vi "Demo HAL Tester v2.vi"() -> ()   [LabVIEW 2014]
uses:
  <vilib>/Utility/miscctls.llb/LVPointTypeDef.ctl
  <vilib>/Utility/miscctls.llb/LVRectTypeDef.ctl
  Typedefs/Driver Data.ctl
  Typedefs/HW Data.ctl
  TypeDefs/HAL Config Data.ctl
  DriverMasterSync/build/DriverMasterSync.lvlibp/Modules/HAL/DriverMasterSync/DriverMasterSyncClass/DriverMasterSync.lvclass
  DriverMasterAsync/builds/DriverMasterAsync.lvlibp/Modules/HAL/DriverMasterAsync/DriverMasterAsyncClass/DriverMasterAsync.lvclass
  <vilib>/Utility/miscctls.llb/LVRangeTypeDef.ctl
  APIs/Message Queue/Enqueue Message (Single).vi
  APIs/Message Queue/WINFAS 2 Message Queue.lvlib
  APIs/Data Queue/WINFAS 2 Data Queue.lvlib
  HWSyncLoop/HWSyncLoop.lvlib
  HWAsyncLoop/HWAsyncLoop.lvlib
  <vilib>/Utility/file.llb/Write To Spreadsheet File (string).vi
  <vilib>/Utility/file.llb/Read From Spreadsheet File (string).vi
  <vilib>/Utility/LVLibp/NI_PackedLibraryUtility.lvlib
panel:
  out "Enable Waveforms":u32
  out "HW Position":i32
  out "Display Tab":enum32{"Splash", "Sync", "Async"}(tab)
  out "Driver Name Sync 2":string
  out "Mensajes para Usuario (Síncronos)":string
  out "Sync DI":bool[][](array[boolean])
  out "Sync DO":bool[][](array[boolean])
  out "Encoder":sgl caption="Encoder:" format="%.1f"
  in  "Escala en mm:":enum32{"x0.25", "x0.5", "x1", "x2"}(radio)=enum."x1"
  out "Tabla TDX":string[][](table)
  out "Waveform Graph":sgl[][](graph)
  out "Mensajes para el usuario (Asíncronos)":string
  out "Tabla Med Async":string[][](table)
  out "Status Bar":string
  out "Command Tab":enum32{"Configuración", "Comandos"}(tab)
  in  "Descripción":string
  in  "Open Cfg":bool
  in  "Save Cfg":bool
  in  "New Cfg":bool
  in  "Driver Tree":string(tree)
  in  "HAL Activate":bool
  in  "Driver Unload":bool
  out "Last Mod":string caption="Última modificación:"
  out "Cfg Driver Name":string caption="Nombre:"
  in  "Cfg Panel Open":bool
  in  "Driver Load":bool
  in  "Dispositivos Conectados":i32(listbox)
  out "Sync/Async CMD":enum32{"Sync", "Async"}(tab)
  out "Estado:":string
  in  "Sync ACQ Start":bool
  in  "Output Control":bool[][](array[boolean])
  in  "Write Digital Out":bool
  in  "Zero Encoder":bool
  out "Driver Name Sync":string
  in  "Async ACQ":bool
  in  "Async Zero":bool
  in  "Async Action 2":bool
  in  "Async Action 1":bool
  out "Driver Name Async":string
  in  "HAL Deactivate":bool
  # "INSTRUCCIONES DE USO\n\n- Panel Configuración-\n1. Crear Nuevo Configuración o Abrir una ya existente (Los archivos de configuración tiene extensión \".config\"; Por ej \"CAP 16T.config\"). Puede guardar  sus propias\nconfiguraciones con el botón Guardar\n\n- Panel Driver -\n1. En la lista desplegable se pueden visualizar y seleccionar los 5 Procesos Síncronos (Sync#) y los 10 Procesos Asíncronos (Async#),\ncon su respectivo driver cargado (Por ej \"CAP-USB-1.lvlibp\")\n2. Una vez seleccionado un Proceso se puede cargar un Driver en el mismo mediante el boton \"\"Cargar Nuevo...\"\n3. Para acceder a su panel de configuración presione \"Configuración...\"\n4. Para eliminar le Driver cargado del proceso seleccionado presione \"Eliminar\"\n\n- CONECTAR -\n1. Una vez definida la configuración de Drivers que uno desea, al presionar \"Conectar >\" se establecerán conexiones con todos los dispositivos elegidos y se comenzará el proceso de\nadquisición en Auto-Refresh de los procesos Síncronos. VERIFIQUE QUE TODO EL CABLEADO ESTÉ CORRECTO, sino la aplicación devolverá error.\n\n- Panel Dispositivos Conectados -\n1. Una vez conectados los dispositivos se podrá seleccionar cada Dispositivo que esté funcionando y monitorear sus valores de adquisición, como así también darle comandos \npara que adquiera más datos, realice mediciones, escriba el encoder en Cero,escriba y lea salidas, etc.\n\n- DESCONECTAR -\n1. Una vez que desee terminar con la adquisición, debe presionar \"Desconectar >\". ASEGURESE QUE NINGÚN DISPOSITIVO ESTE EN ESTADO DE MEDICIÓN,\nsino la aplicación devolverá error."
  # "Medición de Transductores (TODOS)"
  # "Encoder y Entradas/Salidas Digitales"
  # "Entradas"
  # "1      2      3      4      5      6      7      8      9     10    11    12    13    14    15    16"
  # "17    18    19    20    21    22    23    24    25    26    27    28    29    30    31    32"
  # "Salidas"
  # "1      2      3      4      5      6      7      8      9     10    11    12    13    14    15    16"
  # "17    18    19    20    21    22    23    24    25    26    27    28    29    30    31    32"
  # "Valores medidos (Asíncronos)"
  # "Configuración"
  # "Conecta todos los dispositivos y comienza\nel ciclo de prueba"
  # "Driver Seleccionado"
  # "Comandos"
  # "(Dispositivo Midiendo = subrayado)"
  # "Medición"
  # "(Solo se permite de a un dispositivo por vez)"
  # "Salidas Digitales"
  # "Seleccione los estados de las salidas y presione\n\"Escribir Salidas\" para escribir el puerto entero"
  # "1      2      3      4      5      6      7      8      9     10    11    12    13    14    15    16"
  # "17    18    19    20    21    22    23    24    25    26    27    28    29    30    31    32"
  # "Encoder"
  # "Pone al encoder en valor 0 (Cero)"
  # "Acción"
  # "Medición"
  # "Realizo una medición asíncrona"
  # "Realiza Acción 1"
  # "Poner en Cero el Dispositivo"
  # "Realiza Acción 2"
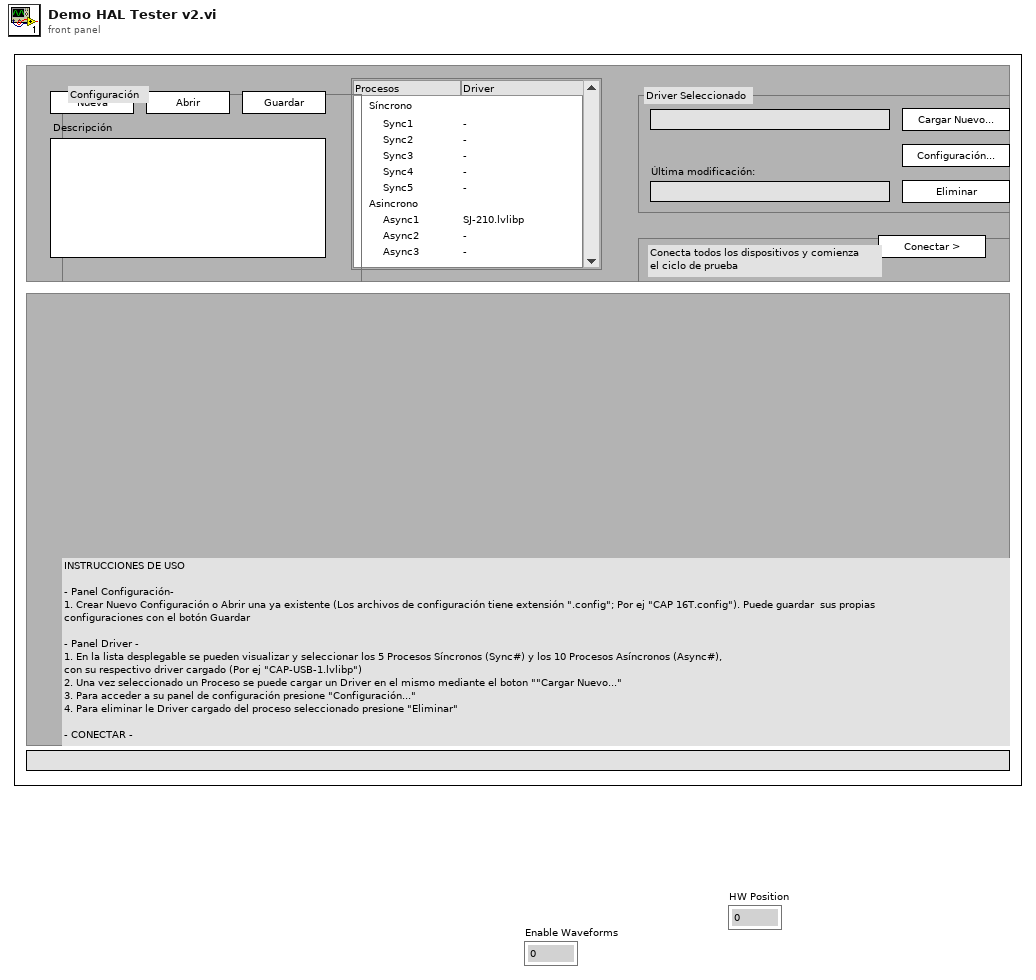
[diagram p1: front panel]
types:
  T1 = typedef "HAL Config Data.ctl" = cluster{"HWSync Index":u32, "Driver Name":string, "Channel Mask":u64}
  T2 = typedef "HW Data.ctl" = cluster{"Driver Name":string, "Sincrono?":bool, "HW Position":i32, "Busy?":bool}
  T3 = enum8{"Enabled", "Disabled", "Disabled and Grayed Out"}
  T4 = typedef "Driver Data.ctl" = cluster{"Dirección de Driver":path, "Config Data":variant}
  T5 = typedef "LVRectTypeDef.ctl" = cluster{"Left":i16, "Top":i16, "Right":i16, "Bottom":i16}
  T6 = typedef "LVPointTypeDef.ctl" = cluster{"Horizontal":i16, "Vertical":i16}
  T7 = typedef "WINFAS 2 Message Queue.lvlib/All Message Queues.ctl" = cluster{"CORE":refnum<queue>, "Event UI":refnum<queue>, "Display UI":refnum<queue>, "MATH":refnum<queue>, "SEQ":refnum<queue>, "DB":refnum<queue>, "ERR":refnum<queue>, "HAL":refnum<queue>, "HWSync1":refnum<queue>, "HWSync2":refnum<queue>, "HWSync3":refnum<queue>, "HWSync4":refnum<queue>, "HWSync5":refnum<queue>, "HWAsync1":refnum<queue>, "HWAsync2":refnum<queue>, "HWAsync3":refnum<queue>, "HWAsync4":refnum<queue>, "HWAsync5":refnum<queue>, "HWAsync6":refnum<queue>, "HWAsync7":refnum<queue>, "HWAsync8":refnum<queue>, "HWAsync9":refnum<queue>, "HWAsync10":refnum<queue>}
  T8 = typedef "WINFAS 2 Data Queue.lvlib/All Data Queues Cluster.ctl" = cluster{"Queues":cluster{"ACQ HWSync1":refnum<queue>, "ACQ HWSync2":refnum<queue>, "ACQ HWSync3":refnum<queue>, "ACQ HWSync4":refnum<queue>, "ACQ HWSync5":refnum<queue>}, "Notifiers":cluster{"Control":cluster{"CTRL HWSync1":refnum<notifier>, "CTRL HWSync2":refnum<notifier>, "CTRL HWSync3":refnum<notifier>, "CTRL HWSync4":refnum<notifier>, "CTRL HWSync5":refnum<notifier>}, "Acquisition":cluster{"ACQ HWSync1":refnum<notifier>, "ACQ HWSync2":refnum<notifier>, "ACQ HWSync3":refnum<notifier>, "ACQ HWSync4":refnum<notifier>, "ACQ HWSync5":refnum<notifier>}, "Async":cluster{"ACQ HWAsync1":refnum<notifier>, "ACQ HWAsync2":refnum<notifier>, "ACQ HWAsync3":refnum<notifier>, "ACQ HWAsync4":refnum<notifier>, "ACQ HWAsync5":refnum<notifier>, "ACQ HWAsync6":refnum<notifier>, "ACQ HWAsync7":refnum<notifier>, "ACQ HWAsync8":refnum<notifier>, "ACQ HWAsync9":refnum<notifier>, "ACQ HWAsync10":refnum<notifier>}}}
  T9 = enum16{"open", "replace", "create", "open or create", "replace or create", "replace or create with confirmation"}
  T10 = typedef "LVRangeTypeDef.ctl" = cluster{"Minimum":dbl, "Maximum":dbl, "Increment":dbl, "Minor Increment":dbl, "Start":dbl}
  T11 = cluster{"Dirección de Driver":path, "Config Data":variant}
  T12 = cluster{"Dirección de Driver":path, "Config Data":variant}[]
  T13 = cluster{"ACQ HWSync1":refnum<notifier>, "ACQ HWSync2":refnum<notifier>, "ACQ HWSync3":refnum<notifier>, "ACQ HWSync4":refnum<notifier>, "ACQ HWSync5":refnum<notifier>}
  T14 = cluster{"CTRL HWSync1":refnum<notifier>, "CTRL HWSync2":refnum<notifier>, "CTRL HWSync3":refnum<notifier>, "CTRL HWSync4":refnum<notifier>, "CTRL HWSync5":refnum<notifier>}
  T15 = cluster{"ACQ HWSync1":refnum<queue>, "ACQ HWSync2":refnum<queue>, "ACQ HWSync3":refnum<queue>, "ACQ HWSync4":refnum<queue>, "ACQ HWSync5":refnum<queue>}
  T16 = typedef "WINFAS 2 Data Queue.lvlib/Async Acquisition Data Cluster.ctl" = cluster{"Data":sgl[]}
  T17 = typedef "WINFAS 2 Data Queue.lvlib/Acquisition Data 1 Sample Cluster.ctl" = cluster{"TDX":sgl[], "Encoder":sgl}
  T18 = typedef "WINFAS 2 Data Queue.lvlib/Control Data Cluster.ctl" = cluster{"Encoder":sgl, "DI":bool[], "DO":bool[]}
  T19 = cluster{"HWSync1":refnum<queue>, "HWSync2":refnum<queue>, "HWSync3":refnum<queue>, "HWSync4":refnum<queue>, "HWSync5":refnum<queue>}
  T20 = cluster{"HWAsync1":refnum<queue>, "HWAsync2":refnum<queue>, "HWAsync3":refnum<queue>, "HWAsync4":refnum<queue>, "HWAsync5":refnum<queue>, "HWAsync6":refnum<queue>, "HWAsync7":refnum<queue>, "HWAsync8":refnum<queue>, "HWAsync9":refnum<queue>, "HWAsync10":refnum<queue>}
  T21 = enum32{"invalid app kind", "Development System", "Run Time System", "Student Edition", "Embedded LabVIEW", "Evaluation", "Custom"}
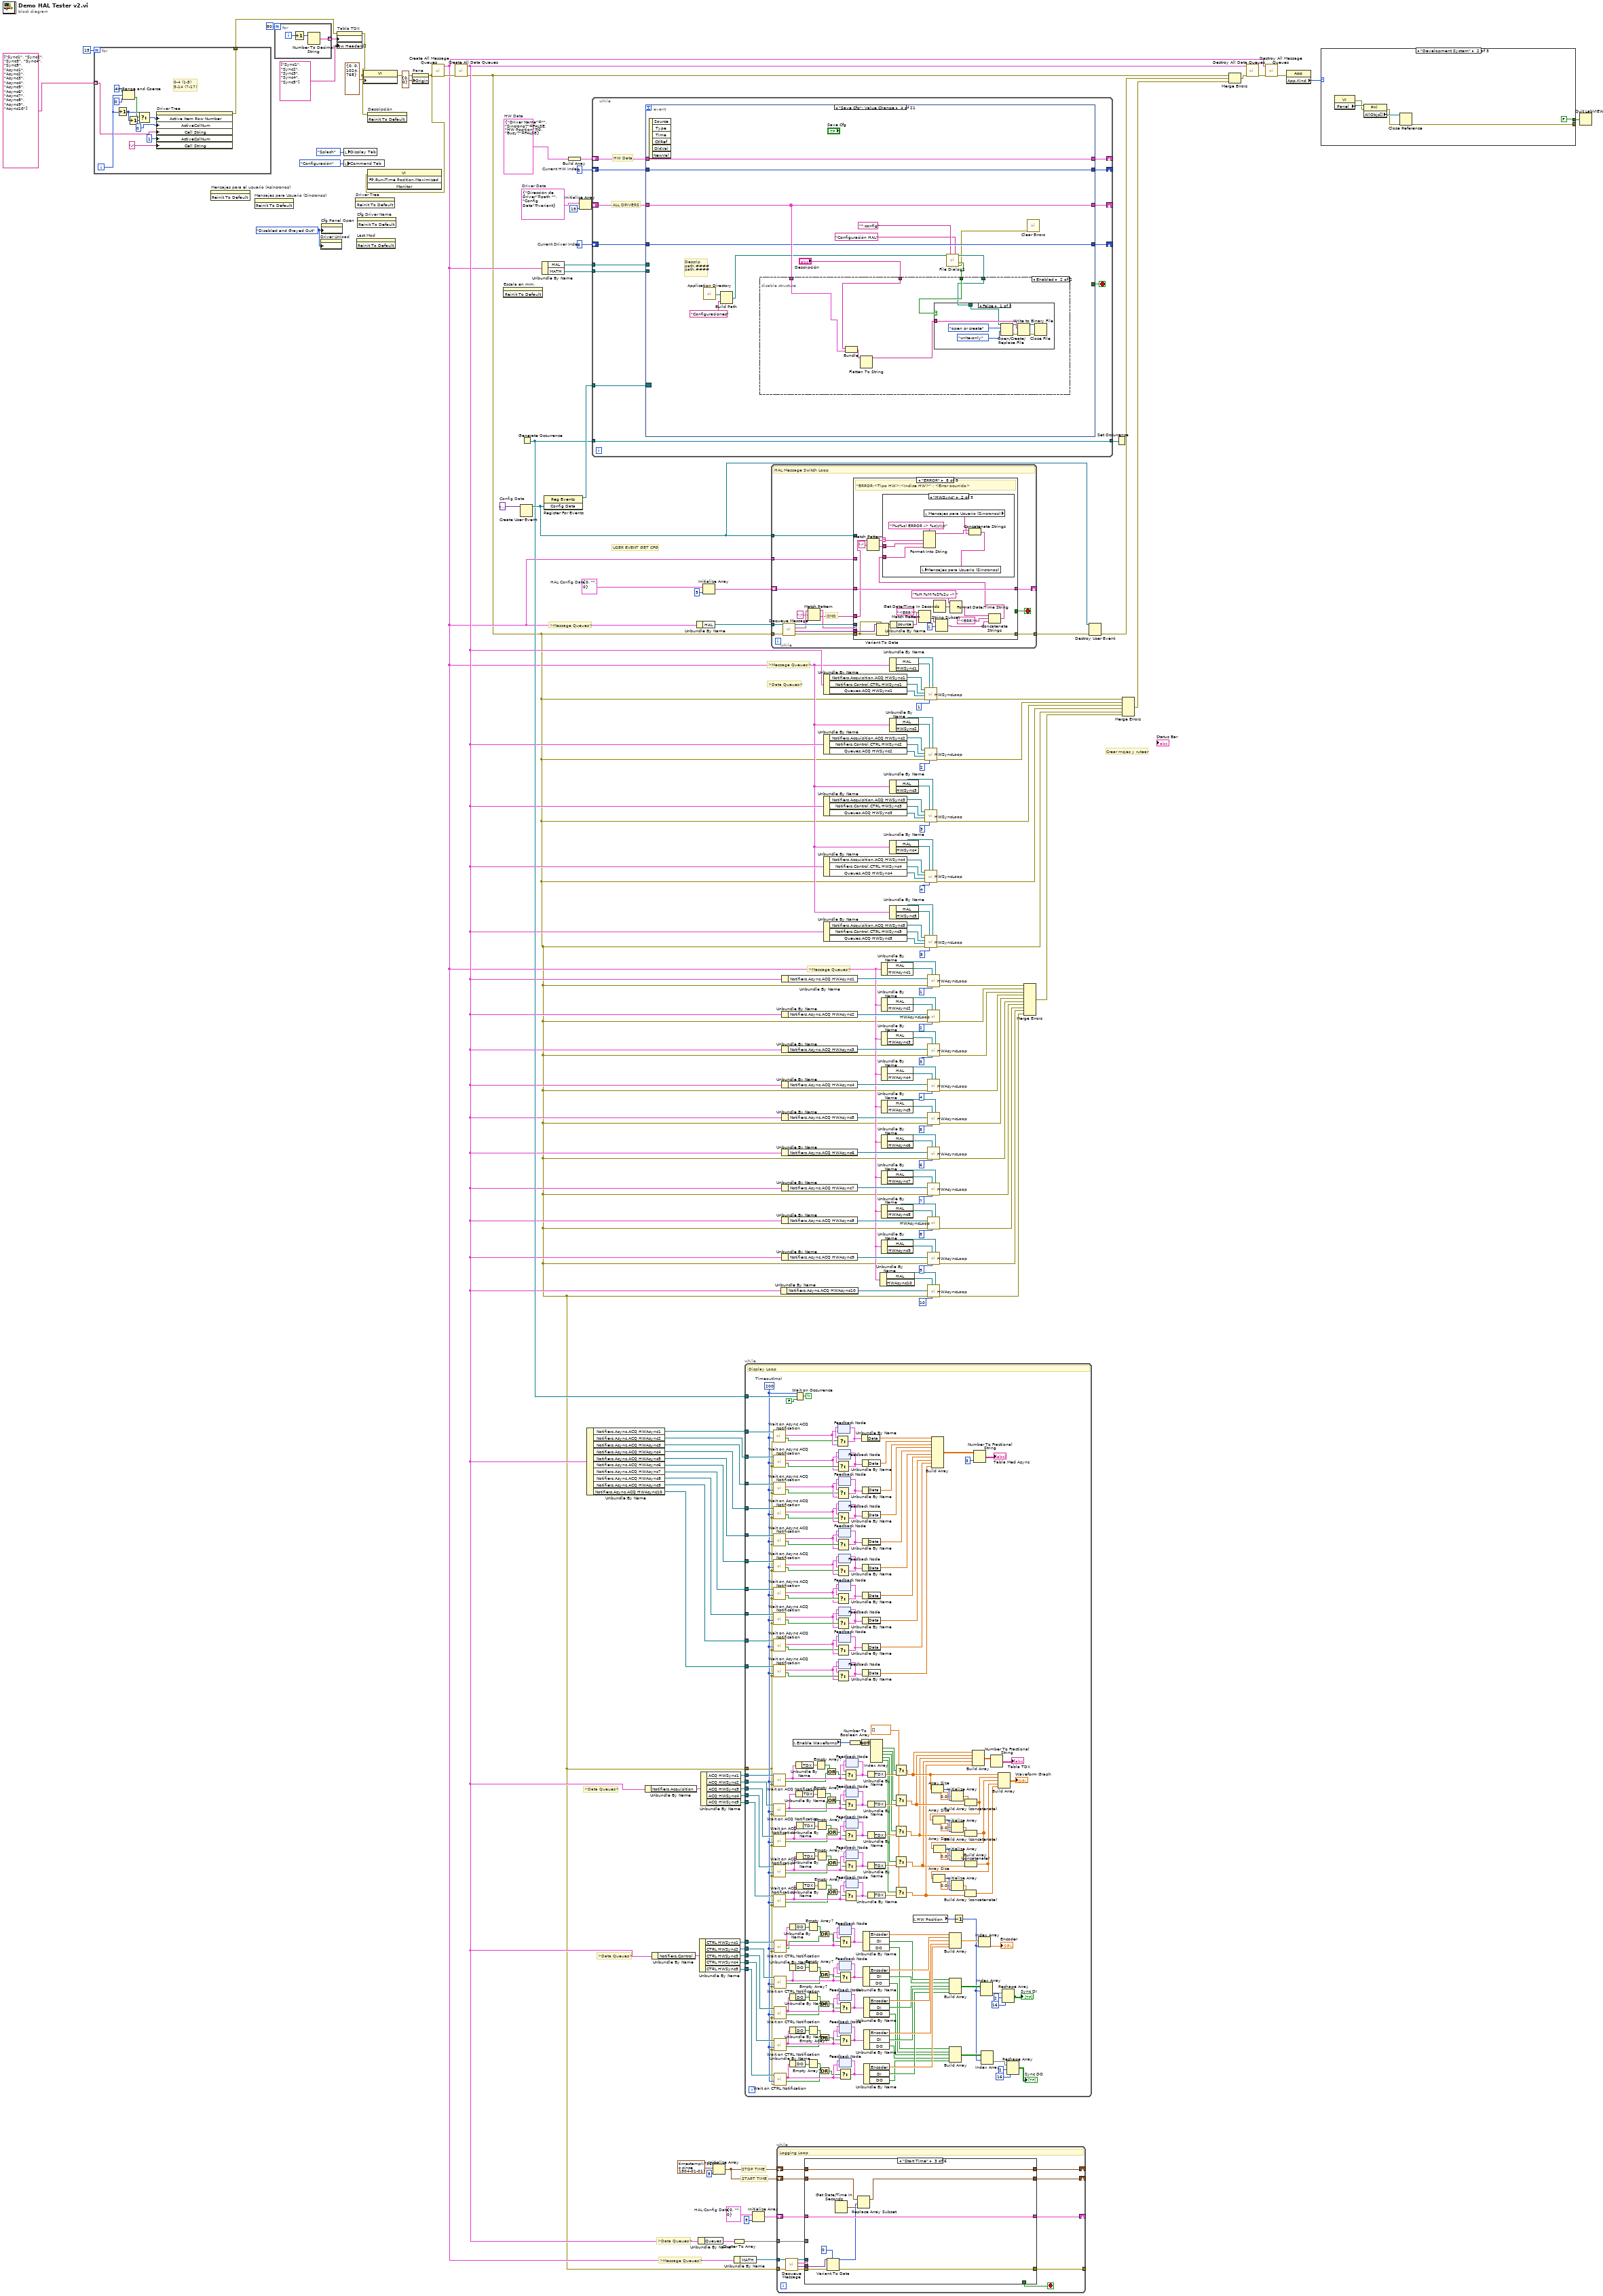
[diagram p0: block diagram]
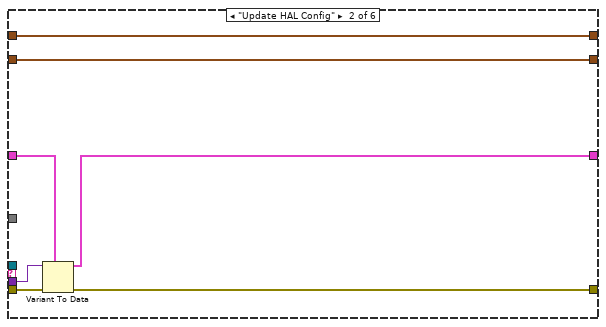
[diagram p3: hidden frame]
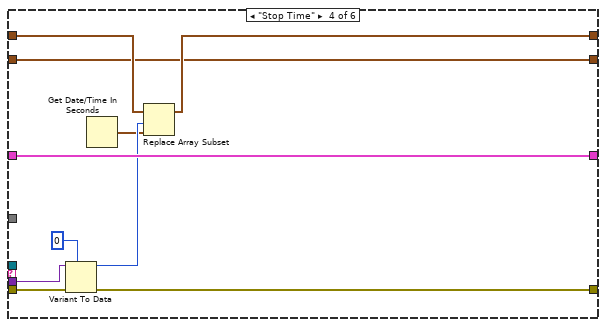
[diagram p4: hidden frame]
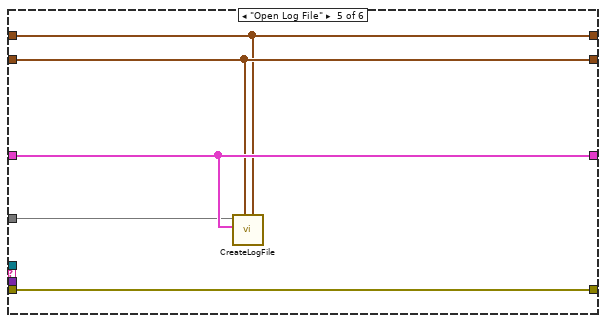
[diagram p5: hidden frame]
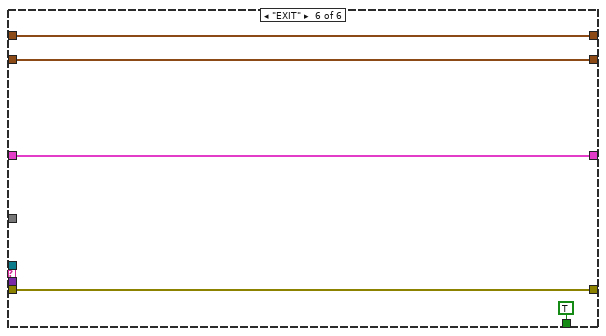
[diagram p6: hidden frame]
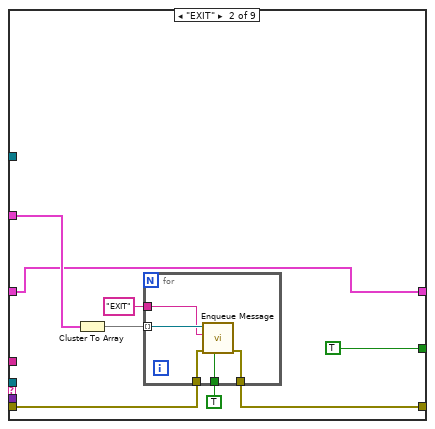
[diagram p8: hidden frame]
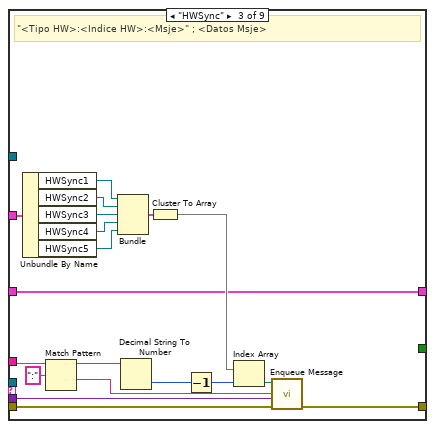
[diagram p9: hidden frame]
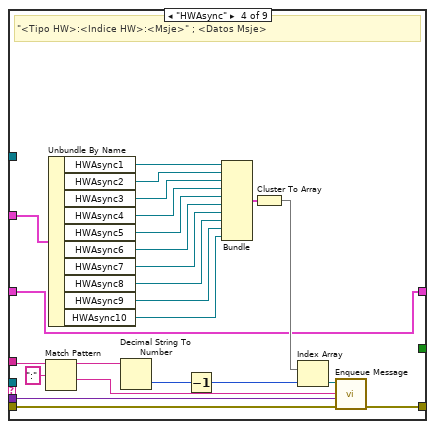
[diagram p10: hidden frame]
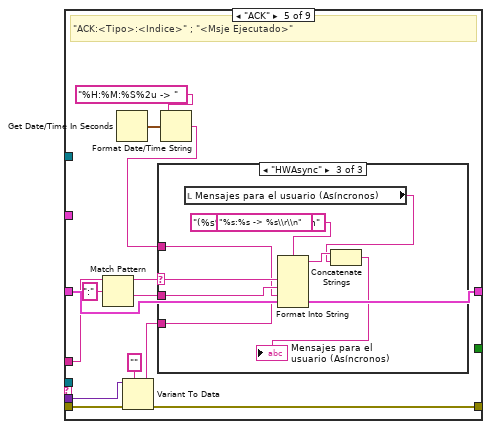
[diagram p11: hidden frame]
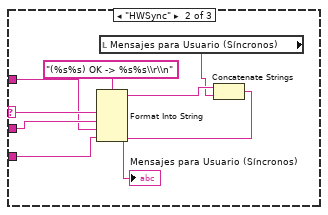
[diagram p13: hidden frame]
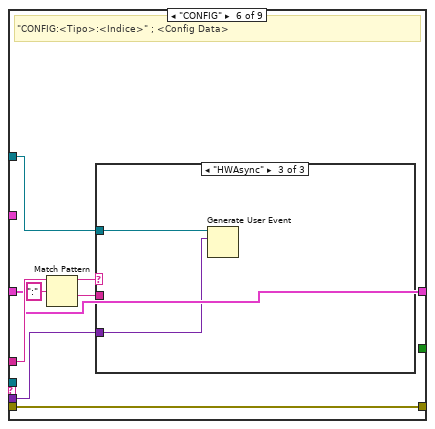
[diagram p14: hidden frame]
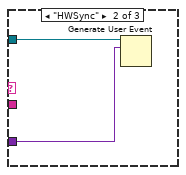
[diagram p16: hidden frame]
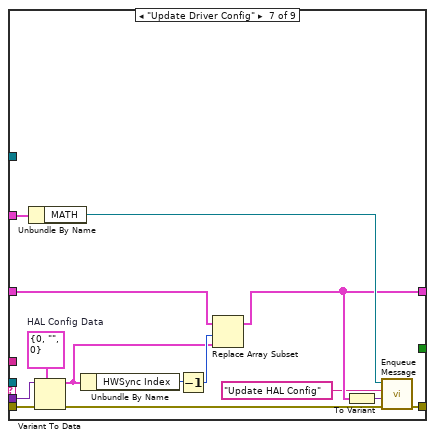
[diagram p17: hidden frame]
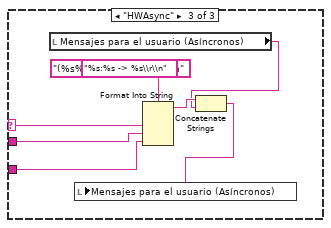
[diagram p19: hidden frame]
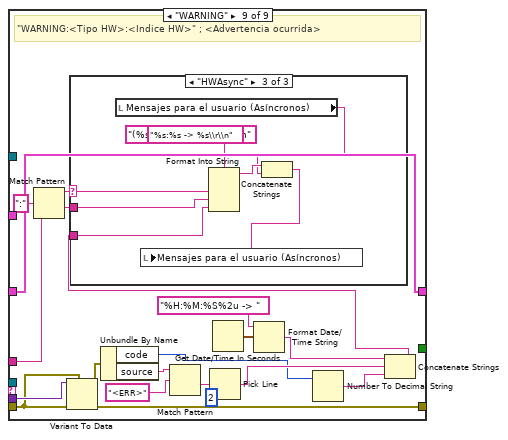
[diagram p20: hidden frame]
diagram:
  w10 = T1 {"HWSync Index"=0, "Driver Name"="", "Channel Mask"=0}  # HAL Config Data
  w41 = T2 {"Driver Name"="", "Sincrono?"=FALSE, "HW Position"=0, "Busy?"=FALSE}  # HW Data
  w42 = 0  # Current HW Index
  w48 = variant  # Config Data
  w49 = T3."Disabled and Grayed Out" ("Disabled")
  w68 = T1 {"HWSync Index"=0, "Driver Name"="", "Channel Mask"=0}  # HAL Config Data
  w152 = 0  # Current Driver Index
  w155 = T4 {"Dirección de Driver"=path "", "Config Data"=variant}  # Driver Data
  # "START TIME"
  # "STOP TIME"
  # ">Data Queues>"
  # ">Message Queues>"
  # ">Data Queues>"
  # ">Data Queues>"
  # "USER EVENT GET CFG"
  # ">Message Queues>"
  # ">Message Queues>"
  # ">Data Queues>"
  # ">Message Queues>"
  # "Crear msjes y rutear"
  n1 = for {
    N: 15 -> [_]
    tunnel: string[] ["Sync1", "Sync2", "Sync3", "Sync4", "Sync5", "Async1", "Async2", "Async3", "Async4", "Async5", "Async6", "Async7", "Async8", "Async9", "Async10"] ("Row Header Strings[]") -> [w164] mode=indexing
    tunnel: [w162] -> w51
    i -> [w168]
    # "0-4 (1-5)\n5-14 (7-17)"
    n2 = Increment(x=w168) -> (x+1=w173:i32)
    n3 = In Range and Coerce(upper limit=4, x=w168, lower limit=0) -> (In Range?=w169:bool)  [unwired: 1 out]
    n4 = Increment(x=w173) -> (x+1=w172:i32)
    n5 = Select(t=w173, s=w169, f=w172) -> (s? t:f=w166:i32)
    n6 = property on="Driver Tree" class="TreeControl (strict)"("Active Item Row Number"=w166, "ActiveColNum"=0 ("Active Cell:Active Column Number"), "Cell String"=w164, "ActiveColNum"=1 ("Active Cell:Active Column Number"), "Cell String"="-" ("Active Cell:String")) -> (error out=w162:errorcluster)  [unwired: 2 in, 1 out]
  }
  n7 = invoke on="Mensajes para el usuario (Asíncronos)" class="Str" method="Reinit To Default"() -> ()  [unwired: 3 in, 3 out]
  n8 = invoke on="Mensajes para Usuario (Síncronos)" class="Str" method="Reinit To Default"() -> ()  [unwired: 3 in, 3 out]
  n9 = for {
    N: 80 -> [_]
    tunnel: [w176] -> w159 mode=indexing
    i -> [w175]
    n10 = Increment(x=w175) -> (x+1=w174:i32)
    n11 = Number To Decimal String(number=w174) -> (decimal integer string=w176:string)  [unwired: 1 in]
  }
  n12 = property on="Driver Unload" class="Bool"("DisabledEnum"=w49) -> ()  [unwired: 2 in, 2 out]
  n13 = property on="Cfg Panel Open" class="Bool"("DisabledEnum"=w49) -> ()  [unwired: 2 in, 2 out]
  n14 = property on="Tabla TDX" class="Tbl (strict)"(error in=w51, "Column Headers[]"=w159, "Row Headers[]"=string[] ["Sync1", "Sync2", "Sync3", "Sync4", "Sync5"] ("Row Header Strings[]")) -> (error out=w50:errorcluster)  [unwired: 1 in, 1 out]
  n15 = local write "Command Tab"(enum32{"Configuración", "Comandos"}."Configuración" ("Command Tab")) -> ()
  n16 = local write "Display Tab"(enum32{"Splash", "Sync", "Async"}."Splash" ("Display Tab")) -> ()
  n17 = invoke on="Driver Tree" class="Tree (strict)" method="Reinit To Default"() -> ()  [unwired: 3 in, 3 out]
  n18 = invoke on="Last Mod" class="Str" method="Reinit To Default"() -> ()  [unwired: 3 in, 3 out]
  n19 = invoke on="Cfg Driver Name" class="Str" method="Reinit To Default"() -> ()  [unwired: 3 in, 3 out]
  n20 = property class="VI"(error in=w50, "Front Panel.WinBounds"=T5 {"Left"=0, "Top"=0, "Right"=1024, "Bottom"=768} ("Front Panel Window:Window Bounds")) -> (error out=w156:errorcluster)  [unwired: 1 in, 1 out]
  n21 = invoke on="Descripción" class="Str" method="Reinit To Default"(error in=w50) -> ()  [unwired: 2 in, 3 out]
  n22 = property on="Pane" class="Pane"(error in=w156, "Origin"=T6 {"Horizontal"=0, "Vertical"=0}) -> (error out=w1:errorcluster)  [unwired: 1 in, 1 out]
  n23 = invoke class="VI" method="FP.Run-Time Position.Maximized"(error in=w1) -> ()  [unwired: 3 in, 4 out]
  n24 = call "Create All Message Queues.vi"("error in (no error)"=w1) -> ("error out"=w151:errorcluster, "Message Queues Out"=w4:T7)  [unwired: 9 in]
  n25 = call "Create All Data Queues.vi"("Error In"=w151) -> ("Error Out"=w3:errorcluster, "WINFAS 2 Data Queue.lvlib:All Data Queues Cluster"=w5:T8)  [unwired: 9 in]
  n26 = invoke on="Escala en mm:" class="RadioBtnsControl (strict)" method="Reinit To Default"() -> ()  [unwired: 3 in, 3 out]
  n27 = Create User Event(user event datatype=w48) -> (user event=w44:refnum<user-event>)  [unwired: 1 in, 1 out]
  n28 = Generate Occurrence() -> (w24:refnum<k4>)
  n29 = Unbundle By Name(w4) -> ("HAL"=w54:refnum<queue>, "MATH"=w2:refnum<queue>)
  n30 = register-events(w44) -> (reference out=w47:refnum<event-registration>)  [unwired: 2 in, 1 out]
  n31 = Build Array(w41) -> (w40:T2[])
  n32 = Initialize Array(w155, 15 ("dimension size")) -> (w153:T4[])
  n33 = Unbundle By Name(w5) -> ("Notifiers.Async.ACQ HWAsync1"=w26:refnum<notifier>, "Notifiers.Async.ACQ HWAsync2"=w23:refnum<notifier>, "Notifiers.Async.ACQ HWAsync3"=w22:refnum<notifier>, "Notifiers.Async.ACQ HWAsync4"=w21:refnum<notifier>, "Notifiers.Async.ACQ HWAsync5"=w20:refnum<notifier>, "Notifiers.Async.ACQ HWAsync6"=w19:refnum<notifier>, "Notifiers.Async.ACQ HWAsync7"=w18:refnum<notifier>, "Notifiers.Async.ACQ HWAsync8"=w17:refnum<notifier>, "Notifiers.Async.ACQ HWAsync9"=w16:refnum<notifier>, "Notifiers.Async.ACQ HWAsync10"=w15:refnum<notifier>)
  n34 = while {
    shift-right: [w187] -> _
    shift-left: w152 -> [w188]
    shift-right: [w186] -> _
    shift-left: w153 -> [w189]
    tunnel: w54 -> [w185]
    tunnel: w47 -> [w184]
    shift-right: [w181] -> _
    shift-left: w40 -> [w182]
    shift-right: [w180] -> _
    shift-left: w42 -> [w183]
    tunnel: w24 -> [w179]
    tunnel: [w179] -> w25
    tunnel: w2 -> [w178]
    stop <- w177 stop-if-true
    # "HW Data"
    # "ALL DRIVERS"
    n35 = event shown="[3] \"Save Cfg\": Value Change" {
      selector: w184 -> [_ _ _ _ _ _ _ _ _ _ _ _ _ _ _ _ _ _ _ _ _]
      dyn-events: _ -> [_ _ _ _ _ _ _ _ _ _ _ _ _ _ _ _ _ _ _ _ _]
      timeout: _ -> [_ _ _ _ _ _ _ _ _ _ _ _ _ _ _ _ _ _ _ _ _]
      tunnel: w189 -> [w193 w199 w244 w350 w401 w433 w513 w524 w528 w538 w559 w622 w654 w681 w736 w779 w794 w805 w816 w827 w838]
      tunnel: w188 -> [w192 w206 w238 w349 _ w424 w514 w517 w530 w539 w561 w623 w655 w682 w737 w780 w795 w806 w817 w828 w839]
      tunnel: [w192 w205 w239 w349 w402 w424 w514 w517 w530 w539 w561 w623 w655 w682 w737 w780 w795 w806 w817 w828 w839] -> w187
      tunnel: [w193 w207 w243 w350 w401 w432 w513 w524 w527 w537 w559 w622 w654 w681 w736 w779 w794 w805 w816 w827 w838] -> w186
      tunnel: w185 -> [_ w203 w240 _ _ w437 w507 w521 _ w551 w560 w621 _ _ w720 w771 w783 w799 w810 w821 w832]
      tunnel: w183 -> [w190 w194 w235 w343 w393 w422 w511 w515 w525 w534 w558 w620 w652 _ w724 w772 w792 w800 w811 w822 w833]
      tunnel: w182 -> [w191 w195 w236 w344 w394 w423 w512 w516 w526 w535 w552 w619 w653 w662 w719 w773 w793 w801 w812 w823 w834]
      tunnel: [w191 w195 w236 w344 w394 w423 w512 w516 w526 w535 w557 T2[] [] w653 w662 w727 w773 w793 w801 w812 w823 w834] -> w181
      tunnel: [w190 w194 w235 w343 w393 w422 w511 w515 w525 w534 w558 w620 w652 "Dispositivos Conectados" w724 w772 w792 w800 w811 w822 w833] -> w180
      tunnel: w178 -> [_ _ _ _ _ _ w506 _ _ _ _ _ _ _ w717 _ _ _ _ _ _]
      tunnel: [_ _ _ _ _ _ w505 _ _ _ _ _ _ _ _ _ _ _ _ _ _] -> w177
      event Timeout {
        n36 = event-data() -> ()  [unwired: 1 in, 3 out]
      }
      event "New Cfg": Value Change {
        w201 = T11 {"Dirección de Driver"=path "", "Config Data"=variant}  # Driver Data
        n37 = event-data() -> ()  [unwired: 1 in, 6 out]
        n38 = Initialize Array(w201, 15 ("dimension size")) -> (w200:T12)
        n39 = Flatten To String(anything=w200) -> (data string=w197:string)  [unwired: 3 in, 2 out]
        n40 = Flatten To String(anything=w199) -> (data string=w198:string)  [unwired: 3 in, 2 out]
        n41 = Not Equal?(x=w198, y=w197) -> (x != y?=w196:bool)
        n42 = case "Algún Driver cargado?" shown="True" w196 {
          tunnel: [TRUE ("T button?") w210] -> w204
          frame False {
          }
          frame True {
            n43 = Two Button Dialog(message="Desea crear una nueva configuración?\n(Se descargarán todos los Drivers cargados)") -> (T button?=w210:bool)  [unwired: 2 in]
          }
        }
        n44 = case shown="True" w204 {
          tunnel: [w212 w218] -> w207
          tunnel: w199 -> [w212 _]
          tunnel: w206 -> [w211 _]
          tunnel: [w211 0] -> w205
          tunnel: w203 -> [_ w216]
          frame False {
          }
          frame True {
            w214 = T3."Disabled and Grayed Out" ("Disabled")
            n45 = invoke on="Driver Tree" class="Tree (strict)" method="Reinit To Default"() -> ()  [unwired: 3 in, 3 out]
            n46 = invoke on="Cfg Driver Name" class="Str" method="Reinit To Default"() -> ()  [unwired: 3 in, 3 out]
            n47 = invoke on="Last Mod" class="Str" method="Reinit To Default"() -> ()  [unwired: 3 in, 3 out]
            n48 = invoke on="Descripción" class="Str" method="Reinit To Default"() -> ()  [unwired: 3 in, 3 out]
            n49 = for {
              N: 15 -> [_]
              tunnel: w216 -> [w228]
              i -> [w221]
              n50 = call "Driver Parse CMD.vi"("Cmd String"="UNLOAD", "Current Driver Index"=w221) -> ("resulting string"=w229:string)  [unwired: 9 in]
              n51 = Increment(x=w221) -> (x+1=w226:i32)
              n52 = In Range and Coerce(upper limit=4, x=w221, lower limit=0) -> (In Range?=w222:bool)  [unwired: 1 out]
              n53 = call-poly "Enqueue Message.vi"("Message"=w229, "Message Queue"=w228) -> ()  [unwired: 8 in, 2 out]
              n54 = Increment(x=w226) -> (x+1=w225:i32)
              n55 = Select(t=w226, s=w222, f=w225) -> (s? t:f=w227:i32)
              n56 = property on="Driver Tree" class="TreeControl (strict)"("Active Item Row Number"=w227, "Cell String"="-" ("Active Cell:String")) -> ()  [unwired: 2 in, 2 out]
            }
            n57 = property on="Driver Unload" class="Bool"("DisabledEnum"=w214) -> ()  [unwired: 2 in, 2 out]
            n58 = property on="Cfg Panel Open" class="Bool"("DisabledEnum"=w214) -> ()  [unwired: 2 in, 2 out]
            n59 = Initialize Array(T4 {"Dirección de Driver"=path "", "Config Data"=variant} ("Driver Data"), 15 ("dimension size")) -> (w218:T4[])
          }
        }
      }
      event "Open Cfg": Value Change {
        n60 = event-data() -> ()  [unwired: 1 in, 6 out]
        n61 = call <vilib>:"Application Directory.vi"() -> ("Application Directory"=w234:path)
        n62 = Build Path(base path=w234, name or relative path="Configuraciones") -> (appended path=w233:path)
        n63 = call "File Dialog"("start path"=w233, "pattern (all files)"="*.config", "pattern label"="Configuración HAL") -> ("selected path"=w245:path, "cancelled"=w231:bool, "error out"=w237:errorcluster)  [unwired: 9 in, 1 out]
        n64 = call <vilib>:"Clear Errors.vi"("error in (no error)"=w237) -> ()  [unwired: 5 in, 2 out]
        n65 = case shown="False" w231 {
          tunnel: w245 -> [w252 _]
          tunnel: w244 -> [w251 w339]
          tunnel: [w246 w339] -> w243
          tunnel: w240 -> [w250 _]
          tunnel: [0 w338] -> w239
          tunnel: w238 -> [_ w338]
          frame False {
            w249 = T3."Disabled and Grayed Out" ("Disabled")
            n66 = disable-structure shown="Enabled" {
              disable-tunnel: w252 -> [w267 w300]
              disable-tunnel: w251 -> [w266 w293]
              disable-tunnel: [w255 w299] -> w247
              disable-tunnel: [w254 w292] -> w246
              frame Disabled {
                n67 = disable-structure shown="Enabled" {
                  disable-tunnel: w267 -> [w270 w273]
                  disable-tunnel: [w268 w271] -> w253
                  frame Disabled {
                    n68 = call-poly <vilib>:"Read From Spreadsheet File.vi"("delimiter (\\t)"="," ("delimiter (\\t)"), "file path (dialog if empty)"=w270) -> ("all rows"=w268:string[][])  [unwired: 5 in, 4 out]
                  }
                  frame Enabled {
                    n69 = Open/Create/Replace File(file path (use dialog)=w273, operation (0:open)=T9."open", access (0:read/write)=enum16{"read/write", "read-only", "write-only"}."read-only") -> (refnum out=w276:refnum<file>, error out=w278:errorcluster)  [unwired: 3 in, 1 out]
                    n70 = Read from Binary File(5:string[][] [], 8:w278, 11:w276) -> (0:w279:errorcluster, 2:w271:string[][], 3:w277:refnum<file>)  [unwired: 3 in, 1 out]
                    n71 = Close File(refnum=w277, error in=w279) -> ()  [unwired: 2 out]
                  }
                }
                n72 = Array Subset(array=w253, index (row)=0 ("index"), length (row)=15 ("length"), index (col)=0 ("index"), length (col)=2 ("length")) -> (w261:string[][])
                n73 = for {
                  tunnel: w266 -> [w289] mode=indexing
                  tunnel: [w285] -> w254 mode=indexing
                  tunnel: w261 -> [w284] mode=indexing
                  n74 = Index Array(array=w284) -> (element #1=w290:string, element #2=w283:string)  [unwired: 2 in]
                  n75 = String To Path(string=w290) -> (path=w288:path)
                  n76 = Unflatten From String(type=variant, binary string=w283) -> (value=w287:variant)  [unwired: 3 in, 2 out]
                  n77 = Bundle By Name(cluster=w289, "Dirección de Driver"=w288, "Config Data"=w287) -> (w285:T4)
                }
                n78 = Array Subset(array=w253, index (row)=15 ("index"), index (col)=0 ("index"), length (col)=2 ("length")) -> (w257:string[][])  [unwired: 1 in]
                n79 = for {
                  tunnel: w257 -> [w282] mode=indexing
                  tunnel: [w280] -> w256 mode=indexing
                  n80 = Concatenate Strings(w282, "\r\n") -> (w280:string)
                }
                n81 = Concatenate Strings(w256) -> (w255:string)
              }
              frame Enabled {
                n82 = Bundle("", w293) -> (w295:cluster{string, T4[]})  [unwired: 1 in]
                n83 = Open/Create/Replace File(file path (use dialog)=w300, operation (0:open)=T9."open", access (0:read/write)=enum16{"read/write", "read-only", "write-only"}."read-only") -> (refnum out=w304:refnum<file>, error out=w302:errorcluster)  [unwired: 3 in, 1 out]
                n84 = Read from Binary File(5:"", 8:w302, 11:w304) -> (0:w301:errorcluster, 2:w296:string, 3:w303:refnum<file>)  [unwired: 3 in, 1 out]
                n85 = Unflatten From String(type=w295, binary string=w296) -> (value=w294:cluster{string, T4[]})  [unwired: 3 in, 2 out]
                n86 = Close File(refnum=w303, error in=w301) -> (error out=w297:errorcluster)  [unwired: 1 out]
                n87 = call <vilib>:"Clear Errors.vi"("error in (no error)"=w297) -> ()  [unwired: 5 in, 2 out]
                n88 = Unbundle(w294) -> (w299:string, w292:T4[])
              }
            }
            n89 = for {
              tunnel: w250 -> [w320]
              tunnel: w246 -> [w318] mode=indexing
              i -> [w309]
              n90 = call "Driver Parse CMD.vi"("Cmd String"="UNLOAD", "Current Driver Index"=w309) -> ("resulting string"=w321:string)  [unwired: 9 in]
              n91 = Unbundle By Name(w318) -> ("Dirección de Driver"=w316:path, "Config Data"=w307:variant)
              n92 = call-poly "Enqueue Message.vi"("Message"=w321, "Message Queue"=w320) -> ("dup Message Queue"=w319:refnum<queue>)  [unwired: 8 in, 1 out]
              n93 = call <vilib>:"Is Path and Not Empty.vi"("path"=w316) -> ("Is Path and Not Empty?"=w317:bool)  [unwired: 4 in]
              n94 = case shown="True" w317 {
                tunnel: w319 -> [_ w334]
                tunnel: w316 -> [_ w333]
                tunnel: w309 -> [_ w324]
                tunnel: ["-" ("name") w332] -> w308
                tunnel: w307 -> [_ w329]
                frame False {
                }
                frame True {
                  n95 = Strip Path(path=w333) -> (name=w332:string)  [unwired: 1 out]
                  n96 = call "Driver Parse CMD.vi"("Cmd String"="LOAD", "Current Driver Index"=w324) -> ("resulting string"=w337:string)  [unwired: 9 in]
                  n97 = To Variant(anything=w333) -> (Variant=w336:variant)
                  n98 = call-poly "Enqueue Message.vi"("Message Data"=w336, "Message"=w337, "Message Queue"=w334) -> ("dup Message Queue"=w326:refnum<queue>)  [unwired: 7 in, 1 out]
                  n99 = call "Driver Parse CMD.vi"("Cmd String"="DRIVER INIT", "Current Driver Index"=w324) -> ("resulting string"=w327:string)  [unwired: 9 in]
                  n100 = call-poly "Enqueue Message.vi"("Message"=w327, "Message Queue"=w326) -> ("dup Message Queue"=w325:refnum<queue>)  [unwired: 8 in, 1 out]
                  n101 = call "Driver Parse CMD.vi"("Cmd String"="Config:Set", "Current Driver Index"=w324) -> ("resulting string"=w331:string)  [unwired: 9 in]
                  n102 = call-poly "Enqueue Message.vi"("Message Data"=w329, "Message"=w331, "Message Queue"=w325) -> ()  [unwired: 7 in, 2 out]
                }
              }
              n103 = Increment(x=w309) -> (x+1=w314:i32)
              n104 = In Range and Coerce(upper limit=4, x=w309, lower limit=0) -> (In Range?=w310:bool)  [unwired: 1 out]
              n105 = Increment(x=w314) -> (x+1=w313:i32)
              n106 = Select(t=w314, s=w310, f=w313) -> (s? t:f=w315:i32)
              n107 = property on="Driver Tree" class="TreeControl (strict)"("Active Item Row Number"=w315, "Cell String"=w308) -> ()  [unwired: 2 in, 2 out]
            }
            n108 = property on="Cfg Panel Open" class="Bool"("DisabledEnum"=w249) -> ()  [unwired: 2 in, 2 out]
            n109 = property on="Driver Unload" class="Bool"("DisabledEnum"=w249) -> ()  [unwired: 2 in, 2 out]
            n110 = invoke on="Last Mod" class="Str" method="Reinit To Default"() -> ()  [unwired: 3 in, 3 out]
            n111 = invoke on="Driver Tree" class="Tree (strict)" method="Reinit To Default"() -> ()  [unwired: 3 in, 3 out]
            n112 = invoke on="Cfg Driver Name" class="Str" method="Reinit To Default"() -> ()  [unwired: 3 in, 3 out]
            n113 = local write "Descripción"(w247) -> ()
          }
          frame True {
          }
        }
      }
      event "Save Cfg": Value Change {
        # "Descrip\npath,####\npath,####"
        n114 = event-data() -> ()  [unwired: 1 in, 6 out]
        n115 = call <vilib>:"Application Directory.vi"() -> ("Application Directory"=w342:path)
        n116 = Build Path(base path=w342, name or relative path="Configuraciones") -> (appended path=w340:path)
        n117 = call "File Dialog2"("start path"=w340, "pattern (all files)"="*.config", "pattern label"="Configuración HAL") -> ("selected path"=w351:path, "cancelled"=w346:bool, "error out"=w345:errorcluster)  [unwired: 9 in, 1 out]
        n118 = disable-structure shown="Enabled" {
          disable-tunnel: "Descripción" -> [w358 w383]
          disable-tunnel: w351 -> [w356 w382]
          disable-tunnel: w350 -> [w354 w379]
          disable-tunnel: w346 -> [w353 w384]
          frame Disabled {
            n119 = for {
              tunnel: w354 -> [w378] mode=indexing
              tunnel: [w375] -> w359 mode=indexing
              n120 = Unbundle By Name(w378) -> ("Dirección de Driver"=w377:path, "Config Data"=w373:variant)
              n121 = Flatten To String(anything=w373) -> (data string=w374:string)  [unwired: 3 in, 2 out]
              n122 = Path To String(path=w377) -> (string=w376:string)
              n123 = Build Array(w376, w374) -> (w375:string[])
            }
            n124 = Build Array(w358) -> (w357:string[])
            n125 = Build Array (concatenate)(w359, w357) -> (w355:string[][])
            n126 = case shown="False" w353 {
              tunnel: w356 -> [w361 _]
              tunnel: w355 -> [w360 _]
              frame False {
                n127 = disable-structure shown="Enabled" {
                  disable-tunnel: w361 -> [w364 w366]
                  disable-tunnel: w360 -> [w363 w365]
                  frame Disabled {
                    n128 = call-poly <vilib>:"Write To Spreadsheet File.vi"("delimiter (\\t)"="," ("delimiter (\\t)"), "2D data"=w363, "file path (dialog if empty)"=w364) -> ()  [unwired: 5 in, 1 out]
                  }
                  frame Enabled {
                    n129 = Open/Create/Replace File(file path (use dialog)=w366, operation (0:open)=T9."open or create", access (0:read/write)=enum16{"read/write", "read-only", "write-only"}."write-only") -> (refnum out=w370:refnum<file>, error out=w368:errorcluster)  [unwired: 3 in, 1 out]
                    n130 = Write to Binary File(file (use dialog)=w370, data=w365, error in=w368) -> (refnum out=w369:refnum<file>, error out=w367:errorcluster)  [unwired: 3 in, 1 out]
                    n131 = Close File(refnum=w369, error in=w367) -> ()  [unwired: 2 out]
                  }
                }
              }
              frame True {
              }
            }
          }
          frame Enabled {
            n132 = Bundle("Descripción"=w383, w379) -> (w381:cluster{"Descripción":string, T4[]})  [unwired: 1 in]
            n133 = Flatten To String(anything=w381) -> (data string=w380:string)  [unwired: 3 in, 2 out]
            n134 = case shown="False" w384 {
              tunnel: w380 -> [w392 _]
              tunnel: w382 -> [w388 _]
              frame False {
                n135 = Open/Create/Replace File(file path (use dialog)=w388, operation (0:open)=T9."open or create", access (0:read/write)=enum16{"read/write", "read-only", "write-only"}."write-only") -> (refnum out=w389:refnum<file>, error out=w386:errorcluster)  [unwired: 3 in, 1 out]
                n136 = Write to Binary File(file (use dialog)=w389, data=w392, error in=w386) -> (refnum out=w387:refnum<file>, error out=w385:errorcluster)  [unwired: 3 in, 1 out]
                n137 = Close File(refnum=w387, error in=w385) -> ()  [unwired: 2 out]
              }
              frame True {
              }
            }
          }
        }
        n138 = call <vilib>:"Clear Errors.vi"("error in (no error)"=w345) -> ()  [unwired: 5 in, 2 out]
      }
      event "Driver Tree": Value Change {
        # "Selector de CURRENT DRIVER"
        # "Selector de HW"
        n139 = event-data() -> ()  [unwired: 1 in, 6 out]
        n140 = property on="Driver Tree" class="TreeControl (strict)"("Active Item Tag"="Driver Tree") -> ("Active Item Row Number"=w404:i32)  [unwired: 2 in, 2 out]
        n141 = Decrement(x=w404) -> (x-1=w405:i32)
        n142 = Greater?(x=w404, y=5) -> (0:w406:bool)
        n143 = Select(t=w405, s=w406, f=w404) -> (s? t:f=w403:i32)
        n144 = Decrement(x=w403) -> (x-1=w402:i32)
        n145 = Index Array(array=w401, index=w402) -> (element=w400:T4)
        n146 = Unbundle By Name(w400) -> ("Dirección de Driver"=w397:path)
        n147 = call <vilib>:"Is Path and Not Empty.vi"("path"=w397) -> ("Is Path and Not Empty?"=w396:bool)  [unwired: 4 in]
        n148 = case shown="True" w396 {
          tunnel: ["" ("date/time string") w413] -> w399
          tunnel: w397 -> [_ w412]
          tunnel: [T3."Disabled and Grayed Out" ("Disabled") T3."Enabled" ("Disabled")] -> w395
          frame False {
          }
          frame True {
            n149 = File/Directory Info(path=w412) -> (last mod=w414:timestamp)  [unwired: 1 in, 6 out]
            n150 = Format Date/Time String(seconds (now)=w414) -> (date/time string=w413:string)  [unwired: 2 in]
          }
        }
        "Last Mod" <- w399
        n151 = Strip Path(path=w397) -> (name=→"Cfg Driver Name":string)  [unwired: 1 out]
        n152 = property on="Driver Unload" class="Bool"("DisabledEnum"=w395) -> ()  [unwired: 2 in, 2 out]
        n153 = property on="Cfg Panel Open" class="Bool"("DisabledEnum"=w395) -> ()  [unwired: 2 in, 2 out]
      }
      event "Driver Load": Value Change {
        n154 = event-data() -> ()  [unwired: 1 in, 6 out]
        n155 = In Range and Coerce(upper limit=4, x=w424, lower limit=0) -> (In Range?=w419:bool)  [unwired: 1 out]
        n156 = call <vilib>:"Application Directory.vi"() -> ("Application Directory"=w418:path)
        n157 = Build Path(base path=w418, name or relative path="Drivers") -> (appended path=w416:path)
        n158 = case shown="True" w419 {
          tunnel: ["Cargar Driver Síncrono" ("button label") "Cargar Driver Asíncrono" ("button label")] -> w430
          tunnel: ["Driver Síncrono" ("pattern label") "Driver Asíncrono" ("pattern label")] -> w429
          tunnel: ["*.lvlibp" ("pattern (all files)") "*.lvlibp" ("pattern (all files)")] -> w428
          tunnel: ["Seleccione Driver Síncrono" ("prompt") "Seleccione Driver Asíncrono" ("prompt")] -> w427
          tunnel: w416 -> [w492 w500]
          tunnel: [w491 w498] -> w415
          frame True {
            n159 = Build Path(base path=w492, name or relative path="Sync") -> (appended path=w491:path)
          }
          frame False {
            n160 = Build Path(base path=w500, name or relative path="Async") -> (appended path=w498:path)
          }
        }
        n161 = call "File Dialog3"("start path"=w415, "prompt"=w427, "button label"=w430, "pattern (all files)"=w428, "pattern label"=w429) -> ("selected path"=w420:path, "cancelled"=w438:bool, "error out"=w431:errorcluster)  [unwired: 7 in, 1 out]
        n162 = case shown="False" w419 {
          tunnel: [w441 w454] -> w421
          tunnel: w420 -> [w440 w453]
          frame True {
            n163 = Strip Path(path=w440) -> (name=w446:string)  [unwired: 1 out]
            n164 = Match Pattern(string=w446, regular expression=".lvlibp") -> (before substring=w445:string)  [unwired: 1 in, 3 out]
            n165 = Format Into String(format string="%s.lvlibp:%s.lvclass", w445, w445) -> (resulting string=w450:string, error out=w442:errorcluster)  [unwired: 2 in]
            n166 = call <vilib>:"Get Exported File Path.vi"("error in (no error)"=w442, "qualified name"=w450, "packed library path"=w440) -> ("error out"=w443:errorcluster, "path"=w451:path)  [unwired: 7 in]
            n167 = call <vilib>:"Get LV Class Default Value.vi"("error in (no error)"=w443, "class path"=w451) -> ("error out"=w444:errorcluster, "object"=w449:refnum<class>)  [unwired: 8 in]
            n168 = To More Specific Class(target class=refnum<class "DriverMasterSync.lvclass"> refnum ("DriverMasterSync.lvlibp:DriverMasterSync.lvclass"), reference=w449, error in=w444) -> (error out=w441:errorcluster)  [unwired: 1 out]
          }
          frame False {
            n169 = Strip Path(path=w453) -> (name=w459:string)  [unwired: 1 out]
            n170 = Match Pattern(string=w459, regular expression=".lvlibp") -> (before substring=w458:string)  [unwired: 1 in, 3 out]
            n171 = Format Into String(format string="%s.lvlibp:%s.lvclass", w458, w458) -> (resulting string=w463:string, error out=w455:errorcluster)  [unwired: 2 in]
            n172 = call <vilib>:"Get Exported File Path.vi"("error in (no error)"=w455, "qualified name"=w463, "packed library path"=w453) -> ("error out"=w456:errorcluster, "path"=w464:path)  [unwired: 7 in]
            n173 = call <vilib>:"Get LV Class Default Value.vi"("error in (no error)"=w456, "class path"=w464) -> ("error out"=w457:errorcluster, "object"=w462:refnum<class>)  [unwired: 8 in]
            n174 = To More Specific Class(target class=refnum<class "DriverMasterAsync.lvclass"> refnum ("DriverMasterAsync.lvlibp:DriverMasterAsync.lvclass"), reference=w462, error in=w457) -> (error out=w454:errorcluster)  [unwired: 1 out]
          }
        }
        n175 = call <vilib>:"Clear Errors.vi"("error in (no error)"=w431) -> ()  [unwired: 5 in, 2 out]
        n176 = Index Array(array=w433) -> (element=w436:T4)  [unwired: 1 in]
        n177 = case shown="Error" w421 {
          selector: w421 -> [_ w490]
          tunnel: w438 -> [w469 _]
          tunnel: w437 -> [w468 _]
          tunnel: [w467 _] -> w435
          tunnel: w424 -> [w466 _]
          tunnel: w420 -> [w465 _]
          frame No Error {
            n178 = case shown="False" w469 {
              tunnel: w466 -> [w472 _]
              tunnel: w465 -> [w475 _]
              tunnel: w468 -> [w485 _]
              tunnel: [w475 path "" ("selected path")] -> w467
              frame False {
                w476 = T3."Enabled" ("Disabled")
                n179 = To Variant(anything=w475) -> (Variant=w487:variant)
                n180 = call "Driver Parse CMD.vi"("Cmd String"="LOAD", "Current Driver Index"=w472) -> ("resulting string"=w486:string)  [unwired: 9 in]
                n181 = Strip Path(path=w475) -> (name=w474:string)  [unwired: 1 out]
                n182 = call-poly "Enqueue Message.vi"("Message Data"=w487, "Message"=w486, "Message Queue"=w485) -> ("dup Message Queue"=w473:refnum<queue>)  [unwired: 7 in, 1 out]
                n183 = File/Directory Info(path=w475) -> (last mod=w477:timestamp)  [unwired: 1 in, 6 out]
                n184 = Increment(x=w472) -> (x+1=w480:i32)
                n185 = In Range and Coerce(upper limit=4, x=w472, lower limit=0) -> (In Range?=w484:bool)  [unwired: 1 out]
                n186 = Increment(x=w480) -> (x+1=w481:i32)
                n187 = Format Date/Time String(seconds (now)=w477) -> (date/time string=w478:string)  [unwired: 2 in]
                n188 = Select(t=w480, s=w484, f=w481) -> (s? t:f=w479:i32)
                n189 = local write "Last Mod"(w478) -> ()
                n190 = call "Driver Parse CMD.vi"("Cmd String"="DRIVER INIT", "Current Driver Index"=w472) -> ("resulting string"=w470:string)  [unwired: 9 in]
                n191 = local write "Cfg Driver Name"(w474) -> ()
                n192 = property on="Driver Tree" class="TreeControl (strict)"("Active Item Row Number"=w479, "Cell String"=w474) -> ()  [unwired: 2 in, 2 out]
                n193 = call-poly "Enqueue Message.vi"("Message"=w470, "Message Queue"=w473) -> ()  [unwired: 8 in, 2 out]
                n194 = property on="Cfg Panel Open" class="Bool"("DisabledEnum"=w476) -> ()  [unwired: 2 in, 2 out]
                n195 = property on="Driver Unload" class="Bool"("DisabledEnum"=w476) -> ()  [unwired: 2 in, 2 out]
              }
              frame True {
              }
            }
          }
          frame Error {
            n196 = call <vilib>:"Clear Errors.vi"("error in (no error)"=w490) -> ()  [unwired: 5 in, 2 out]
            n197 = call "Display Message to User2"() -> ()  [unwired: 10 in, 2 out]
          }
        }
        n198 = Bundle By Name(cluster=w436, "Dirección de Driver"=w435) -> (w434:T4)
        n199 = Replace Array Subset(array=w433, new element=w434, index=w424) -> (w432:T4[])
      }
      event Panel Close? {
        w505 = TRUE ("Discard?")
        w510 = TRUE ("Priority Message? (F)")
        w509 = "EXIT" ("String")
        n200 = event-data() -> ()  [unwired: 1 in, 4 out]
        n201 = call-poly "Enqueue Message.vi"("Priority Message? (F)"=w510, "Message"=w509, "Message Queue"=w506) -> ("error out"=w508:errorcluster)  [unwired: 7 in, 1 out]
        n202 = call-poly "Enqueue Message.vi"("Priority Message? (F)"=w510, "error in (no error)"=w508, "Message"=w509, "Message Queue"=w507) -> ()  [unwired: 6 in, 2 out]
        n203 = event-data("Discard?"=w505) -> ()  [unwired: 1 in, 1 out]
      }
      event "Cfg Panel Open": Value Change {
        w519 = "Config:Get"  # Cmd String
        w523 = "Config"  # Cmd String
        # "#FALTA MSG"
        n204 = event-data() -> ()  [unwired: 1 in, 6 out]
        n205 = call "Driver Parse CMD.vi"("Cmd String"=w523, "Current Driver Index"=w517) -> ("resulting string"=w522:string)  [unwired: 9 in]
        n206 = call-poly "Enqueue Message.vi"("Message"=w522, "Message Queue"=w521) -> ("dup Message Queue"=w518:refnum<queue>)  [unwired: 8 in, 1 out]
        n207 = call "Driver Parse CMD.vi"("Cmd String"=w519, "Current Driver Index"=w517) -> ("resulting string"=w520:string)  [unwired: 9 in]
        n208 = call-poly "Enqueue Message.vi"("Message"=w520, "Message Queue"=w518) -> ()  [unwired: 8 in, 2 out]
      }
      event User Event {
        n209 = event-data() -> ("Config Data"=w529:variant)  [unwired: 1 in]
        n210 = in-place {
          in-place-border: w529 -> [w532]
          n211 = in-place-array #1(w528, w530) -> (w533:T4)
          n212 = Bundle By Name(cluster=w533, "Config Data"=w532) -> (w531:T4)
          n213 = in-place-array #1(w531) -> (w527:T4[])  [unwired: 1 out]
        }
      }
      event "Driver Unload": Value Change {
        w542 = T3."Disabled and Grayed Out" ("Disabled")
        w541 = "" ("Cfg Driver Name")
        # "0-4 (1-5)\n5-14 (7-17)"
        n214 = event-data() -> ()  [unwired: 1 in, 6 out]
        n215 = call "Driver Parse CMD.vi"("Cmd String"="UNLOAD", "Current Driver Index"=w539) -> ("resulting string"=w549:string)  [unwired: 9 in]
        n216 = call-poly "Enqueue Message.vi"("Message"=w549, "Message Queue"=w551) -> ()  [unwired: 8 in, 2 out]
        n217 = Increment(x=w539) -> (x+1=w544:i32)
        n218 = In Range and Coerce(upper limit=4, x=w539, lower limit=0) -> (In Range?=w548:bool)  [unwired: 1 out]
        n219 = Increment(x=w544) -> (x+1=w545:i32)
        n220 = Select(t=w544, s=w548, f=w545) -> (s? t:f=w543:i32)
        n221 = property on="Driver Tree" class="TreeControl (strict)"("Active Item Row Number"=w543, "Cell String"="-" ("Active Cell:String")) -> ()  [unwired: 2 in, 2 out]
        n222 = Replace Array Subset(array=w538, new element=T4 {"Dirección de Driver"=path "", "Config Data"=variant} ("Driver Data"), index=w539) -> (w537:T4[])
        n223 = local write "Cfg Driver Name"(w541) -> ()
        n224 = local write "Last Mod"(w541) -> ()
        n225 = property on="Cfg Panel Open" class="Bool"("DisabledEnum"=w542) -> ()  [unwired: 2 in, 2 out]
        n226 = property on="Driver Unload" class="Bool"("DisabledEnum"=w542) -> ()  [unwired: 2 in, 2 out]
      }
      event "HAL Activate": Value Change {
        n227 = event-data() -> ()  [unwired: 1 in, 6 out]
        n228 = Two Button Dialog(message="Esta seguro que desea conectar todos los dispositivos?", 1:"Cancelar" ("F button name (\"Cancel\")"), 2:"Conectar Dispositivos" ("T button name (\"OK\")")) -> (T button?=w553:bool)
        n229 = case shown="True" w553 {
          tunnel: w560 -> [_ w572]
          tunnel: w559 -> [_ w571]
          tunnel: [w562 w568] -> w557
          tunnel: w552 -> [w562 _]
          frame False {
          }
          frame True {
            n230 = call <vilib>:"Set Busy.vi"() -> ("error out"=w564:errorcluster)  [unwired: 10 in, 1 out]
            n231 = for {
              tunnel: w572 -> [w580]
              tunnel: w571 -> [w583] mode=indexing
              tunnel: [w578] -> w569 mode=indexing if=w576
              tunnel: [w577] -> w568 mode=indexing if=w576
              tunnel: w564 -> [w575]
              tunnel: [w575] -> w563
              i -> [w581]
              n232 = Unbundle By Name(w583) -> ("Dirección de Driver"=w579:path)
              n233 = call <vilib>:"Is Path and Not Empty.vi"("path"=w579) -> ("Is Path and Not Empty?"=w582:bool)  [unwired: 4 in]
              n234 = case shown="False" w582 {
                tunnel: w580 -> [_ w613]
                tunnel: w581 -> [_ w585]
                tunnel: w579 -> [_ w603]
                tunnel: [_ w601] -> w578
                tunnel: [_ TRUE] -> w576
                tunnel: [_ w598] -> w577
                frame False {
                }
                frame True {
                  w599 = T2 {"Driver Name"="", "Sincrono?"=FALSE, "HW Position"=0, "Busy?"=FALSE}  # HW Data
                  n235 = In Range and Coerce(upper limit=4, x=w585, lower limit=0) -> (In Range?=w595:bool)  [unwired: 1 out]
                  n236 = call "Driver Parse CMD.vi"("Cmd String"="Port:Open", "Current Driver Index"=w585) -> ("resulting string"=w615:string)  [unwired: 9 in]
                  n237 = Increment(x=w585) -> (x+1=w610:i32)
                  n238 = Subtract(x=w585, y=4) -> (x-y=w612:i32)
                  n239 = call-poly "Enqueue Message.vi"("Message"=w615, "Message Queue"=w613) -> ("dup Message Queue"=w591:refnum<queue>)  [unwired: 8 in, 1 out]
                  n240 = Select(t=w610, s=w595, f=w612) -> (s? t:f=w596:i32)
                  n241 = Select(t="Sync" ("format string"), s=w595, f="Async" ("format string")) -> (s? t:f=w604:string)
                  n242 = call "Driver Parse CMD.vi"("Cmd String"="Auto-Refresh:Init", "Current Driver Index"=w585) -> ("resulting string"=w592:string)  [unwired: 9 in]
                  n243 = call <vilib>:"Get File Extension.vi"("file"=w603) -> ("filename without extension"=w597:string)  [unwired: 7 in, 3 out]
                  n244 = Format Into String(format string="%s%d", w604, w596) -> (resulting string=w602:string)  [unwired: 2 in, 1 out]
                  n245 = call-poly "Enqueue Message.vi"("Message"=w592, "Message Queue"=w591) -> ("dup Message Queue"=w589:refnum<queue>)  [unwired: 8 in, 1 out]
                  n246 = Build Array(w597, w602) -> (w601:string[])
                  n247 = call "Driver Parse CMD.vi"("Cmd String"="Auto-Refresh:Start", "Current Driver Index"=w585) -> ("resulting string"=w590:string)  [unwired: 9 in]
                  n248 = Bundle By Name(cluster=w599, "Driver Name"=w597, "Sincrono?"=w595, "HW Position"=w596, "Busy?"=FALSE) -> (w598:T2)
                  n249 = call-poly "Enqueue Message.vi"("Message"=w590, "Message Queue"=w589) -> ("dup Message Queue"=w584:refnum<queue>)  [unwired: 8 in, 1 out]
                  n250 = call "Driver Parse CMD.vi"("Cmd String"="Diagnostic:Cycle", "Current Driver Index"=w585) -> ("resulting string"=w587:string)  [unwired: 9 in]
                  n251 = call-poly "Enqueue Message.vi"("Message"=w587, "Message Queue"=w584) -> ()  [unwired: 8 in, 2 out]
                }
              }
            }
            n252 = flat-sequence {
              tunnel: w563 -> [w573]
              tunnel: [w573] -> w565
              frame #0 {
                n253 = Wait (ms)(milliseconds to wait=u32 400) -> ()  [unwired: 1 out]
              }
            }
            n254 = call <vilib>:"Unset Busy.vi"("error in (no error)"=w565) -> ()  [unwired: 10 in, 1 out]
            n255 = property on="Dispositivos Conectados" class="MCListbox (strict)"("Val(Sgnl)"=0 ("Value (Signaling)")) -> (error out=w566:errorcluster)  [unwired: 2 in, 1 out]
            n256 = property on="Dispositivos Conectados" class="MCListbox (strict)"(error in=w566, "ItemNames"=w569) -> ()  [unwired: 1 in, 2 out]
            "Command Tab" <- enum32{"Configuración", "Comandos"}."Comandos" ("Command Tab")
          }
        }
      }
      event "HAL Deactivate": Value Change {
        n257 = event-data() -> ()  [unwired: 1 in, 3 out]
        n258 = for {
          tunnel: w619 -> [w647] mode=indexing
          tunnel: [w646] -> w618 mode=indexing
          n259 = Unbundle By Name(w647) -> ("Busy?"=w646:bool)
        }
        n260 = Or Array Elements(Boolean array=w618) -> (logical OR=w617:bool)
        n261 = case shown="False" w617 {
          tunnel: w622 -> [w629 _]
          tunnel: w621 -> [w628 _]
          frame False {
            n262 = Two Button Dialog(message="Está seguro que desea desconectar los dispositivos?", 1:"Cancelar" ("F button name (\"Cancel\")"), 2:"Desconectar todos" ("T button name (\"OK\")")) -> (T button?=w624:bool)
            n263 = case shown="True" w624 {
              tunnel: w629 -> [_ w633]
              tunnel: w628 -> [_ w632]
              frame False {
              }
              frame True {
                n264 = invoke on="Tabla TDX" class="Tbl (strict)" method="Reinit To Default"() -> ()  [unwired: 3 in, 3 out]
                n265 = invoke on="Mensajes para el usuario (Asíncronos)" class="Str" method="Reinit To Default"() -> ()  [unwired: 3 in, 3 out]
                n266 = invoke on="Mensajes para el usuario (Asíncronos)" class="Str" method="Reinit To Default"() -> ()  [unwired: 3 in, 3 out]
                n267 = invoke on="Mensajes para Usuario (Síncronos)" class="Str" method="Reinit To Default"() -> ()  [unwired: 3 in, 3 out]
                n268 = invoke on="Tabla Med Async" class="Tbl (strict)" method="Reinit To Default"() -> ()  [unwired: 3 in, 3 out]
                n269 = invoke on="Mensajes para Usuario (Síncronos)" class="Str" method="Reinit To Default"() -> ()  [unwired: 3 in, 3 out]
                n270 = invoke on="Waveform Graph" class="WFGraph (strict)" method="Reinit To Default"() -> ()  [unwired: 3 in, 3 out]
                n271 = for {
                  tunnel: w632 -> [w634]
                  tunnel: w633 -> [w638] mode=indexing
                  i -> [w635]
                  n272 = Unbundle By Name(w638) -> ("Dirección de Driver"=w636:path)
                  n273 = call <vilib>:"Is Path and Not Empty.vi"("path"=w636) -> ("Is Path and Not Empty?"=w637:bool)  [unwired: 4 in]
                  n274 = case shown="True" w637 {
                    tunnel: w634 -> [_ w643]
                    tunnel: w635 -> [_ w639]
                    frame False {
                    }
                    frame True {
                      n275 = call "Driver Parse CMD.vi"("Cmd String"="Auto-Refresh:Stop", "Current Driver Index"=w639) -> ("resulting string"=w645:string)  [unwired: 9 in]
                      n276 = call "Driver Parse CMD.vi"("Cmd String"="Port:Close", "Current Driver Index"=w639) -> ("resulting string"=w640:string)  [unwired: 9 in]
                      n277 = call-poly "Enqueue Message.vi"("Message"=w645, "Message Queue"=w643) -> ("dup Message Queue"=w641:refnum<queue>)  [unwired: 8 in, 1 out]
                      n278 = call-poly "Enqueue Message.vi"("Message"=w640, "Message Queue"=w641) -> ()  [unwired: 8 in, 2 out]
                    }
                  }
                }
                n279 = local write "Command Tab"(enum32{"Configuración", "Comandos"}."Configuración" ("Command Tab")) -> ()
                n280 = local write "Display Tab"(enum32{"Splash", "Sync", "Async"}."Splash" ("Display Tab")) -> ()
              }
            }
          }
          frame True {
            n281 = call "Display Message to User"() -> ()  [unwired: 10 in, 2 out]
          }
        }
      }
      event "Escala en mm:": Value Change {
        n282 = event-data() -> ()  [unwired: 1 in, 6 out]
        n283 = case shown="\"x0.5\"" "Escala en mm:" {
          tunnel: [0.25 ("Minimum") 0.5 ("Minimum") 1.0 ("Minimum") 2.0 ("Minimum")] -> w649
          frame "x0.25" {
          }
          frame "x0.5" {
          }
          frame "x1", Default {
          }
          frame "x2" {
          }
        }
        n284 = Multiply(x=w649, y=T10 {"Minimum"=-1.0, "Maximum"=1.0, "Increment"=0.2, "Minor Increment"=0.05, "Start"=-1.0} ("Y Scale.Range")) -> (x*y=w648:T10)
        n285 = property on="Waveform Graph" class="WFGraph (strict)"("YScale.Range"=w648) -> ()  [unwired: 2 in, 2 out]
      }
      event "Dispositivos Conectados": Value Change {
        n286 = event-data() -> ()  [unwired: 1 in, 1 out]
        n287 = for {
          N: 5 -> [_]
          tunnel: w662 -> [w688] mode=indexing
          shift-right: [w685] -> w660
          shift-left: 0 -> [w686]
          n288 = Unbundle By Name(w688) -> ("HW Position"=w684:i32, "Sincrono?"=w687:bool)
          n289 = Decrement(x=w684) -> (x-1=w683:i32)
          n290 = case shown="True" w687 {
            tunnel: w683 -> [_ w693]
            tunnel: w686 -> [w689 w691]
            tunnel: [w689 w690] -> w685
            frame False {
            }
            frame True {
              n291 = Power Of 2(x=w693) -> (2^x=w692:dbl)
              n292 = Add(x=w691, y=w692) -> (x+y=w690:dbl)
            }
          }
        }
        "Enable Waveforms" <- w660
        n293 = for {
          tunnel: w662 -> [w697] mode=indexing
          tunnel: [w696] -> w668 mode=indexing
          n294 = Unbundle By Name(w697) -> ("Busy?"=w696:bool)
        }
        n295 = Index Array(array=w662, index="Dispositivos Conectados") -> (element=w675:T2)
        n296 = Unbundle By Name(w675) -> ("Driver Name"=w671:string, "Sincrono?"=w670:bool, "HW Position"=w666:i32, "Busy?"=w669:bool)
        n297 = Or Array Elements(Boolean array=w668) -> (logical OR=w667:bool)
        n298 = case "Es Sincrono?" shown="True" w670 {
          tunnel: w669 -> [_ w701]
          tunnel: w667 -> [_ w700]
          tunnel: w666 -> [_ w699]
          tunnel: [_ w698] -> w664
          frame False {
          }
          frame True {
            n299 = Exclusive Or(1:w700, 2:w701) -> (0:w702:bool)
            n300 = case "Hay alguno Busy?" shown="False" w702 {
              tunnel: [w711 "Comenzar >" ("format string")] -> w705
              tunnel: w701 -> [w710 _]
              tunnel: [w707 "Monitoreo" ("format string")] -> w704
              tunnel: [T3."Enabled" ("Disabled") T3."Disabled and Grayed Out" ("Disabled")] -> w703
              frame False {
                n301 = Select(t="Midiendo..." ("format string"), s=w710, f="Monitoreo" ("format string")) -> (s? t:f=w707:string)
                n302 = Select(t="Detener X" ("format string"), s=w710, f="Comenzar >" ("format string")) -> (s? t:f=w711:string)
              }
              frame True {
              }
            }
            "Estado:" <- w704
            n303 = property on="Sync ACQ Start" class="Bool"("BoolText.Text"=w705, "DisabledEnum"=w703) -> (error out=w698:errorcluster)  [unwired: 2 in, 1 out]
            "HW Position" <- w699
          }
        }
        n304 = Select(t="Sync" ("format string"), s=w670, f="Async" ("format string")) -> (s? t:f=w672:string)
        n305 = Format Into String(format string="%s (%s%d)", w671, w672, w666) -> (resulting string=→"Driver Name Sync" →"Driver Name Async" →"Driver Name Sync 2":string)  [unwired: 2 in, 1 out]
        n306 = Not(x=w670) -> (.not. x?=w679:bool)
        n307 = Boolean To (0,1)(Boolean=w679) -> (0, 1=w678:i16)
        "Sync/Async CMD" <- w678
        n308 = Increment(x=w678) -> (x+1=→"Display Tab":i16)
        n309 = flat-sequence {
          tunnel: w664 -> [_]
          frame #0 {
            n310 = Wait (ms)(milliseconds to wait=u32 450) -> ()  [unwired: 1 out]
          }
          frame #1 {
            n311 = local read "Sync DO"() -> (w695:bool[][])
            n312 = local write "Output Control"(w695) -> ()
          }
        }
      }
      event "Sync ACQ Start": Value Change {
        n313 = event-data() -> ()  [unwired: 1 in, 4 out]
        n314 = Index Array(array=w719, index=w724) -> (element=w729:T2)
        n315 = Unbundle By Name(w729) -> ("Busy?"=w728:bool)
        n316 = Not(x=w728) -> (.not. x?=w721:bool)
        n317 = Select(t="Midiendo..." ("format string"), s=w721, f="Monitoreo" ("format string")) -> (s? t:f=w735:string)
        n318 = Select(t="Detener X" ("format string"), s=w721, f="Comenzar >" ("format string")) -> (s? t:f=w732:string)
        n319 = Bundle("Current HW Index"=w724, 1) -> (w722:cluster{"Current HW Index":i32, i32})  [unwired: 1 in]
        n320 = Bundle("Current HW Index"=w724, 0) -> (w726:cluster{"Current HW Index":i32, i32})  [unwired: 1 in]
        n321 = local write "Estado:"(w735) -> ()
        n322 = property on="Sync ACQ Start" class="Bool"("BoolText.Text"=w732) -> ()  [unwired: 2 in, 2 out]
        n323 = property on="Dispositivos Conectados" class="MCListbox (strict)"("ActiveCell"=w726, "CellFontUnder"=w721, "ActiveCell"=w722, "CellFontUnder"=w721) -> ()  [unwired: 2 in, 2 out]
        n324 = Bundle By Name(cluster=w729, "Busy?"=w721) -> (w718:T2)
        n325 = case shown="False" w721 {
          tunnel: w720 -> [w753 w767]
          tunnel: w718 -> [w743 w763]
          tunnel: w717 -> [w740 w760]
          frame True {
            n326 = Unbundle By Name(w743) -> ("HW Position"=w754:i32)
            n327 = Decrement(x=w754) -> (x-1=w739:i32)
            n328 = To Variant(anything=w739) -> (Variant=w742:variant)
            n329 = call "Driver Parse CMD.vi"("Cmd String"="Auto-Refresh:Stop", "Current Driver Index"=w739) -> ("resulting string"=w756:string)  [unwired: 9 in]
            n330 = call "Driver Parse CMD.vi"("Cmd String"="Sequence:Init", "Current Driver Index"=w739) -> ("resulting string"=w751:string)  [unwired: 9 in]
            n331 = call "Driver Parse CMD.vi"("Cmd String"="Sequence:Start", "Current Driver Index"=w739) -> ("resulting string"=w749:string)  [unwired: 9 in]
            n332 = call "Driver Parse CMD.vi"("Cmd String"="Diagnostic:Measurement", "Current Driver Index"=w739) -> ("resulting string"=w745:string)  [unwired: 9 in]
            n333 = call-poly "Enqueue Message.vi"("Message"=w756, "Message Queue"=w753) -> ("dup Message Queue"=w750:refnum<queue>)  [unwired: 8 in, 1 out]
            n334 = call-poly "Enqueue Message.vi"("Message"=w751, "Message Queue"=w750) -> ("dup Message Queue"=w747:refnum<queue>)  [unwired: 8 in, 1 out]
            n335 = call-poly "Enqueue Message.vi"("Message"=w749, "Message Queue"=w747) -> ("dup Message Queue"=w744:refnum<queue>)  [unwired: 8 in, 1 out]
            n336 = call-poly "Enqueue Message.vi"("Message"=w745, "Message Queue"=w744) -> ("error out"=w738:errorcluster)  [unwired: 8 in, 1 out]
            n337 = call-poly "Enqueue Message.vi"("error in (no error)"=w738, "Message Data"=w742, "Message"="Start Time", "Message Queue"=w740) -> ()  [unwired: 6 in, 2 out]
          }
          frame False {
            n338 = Unbundle By Name(w763) -> ("HW Position"=w768:i32)
            n339 = Decrement(x=w768) -> (x-1=w759:i32)
            n340 = To Variant(anything=w759) -> (Variant=w761:variant)
            n341 = call "Driver Parse CMD.vi"("Cmd String"="Sequence:Stop", "Current Driver Index"=w759) -> ("resulting string"=w770:string)  [unwired: 9 in]
            n342 = call "Driver Parse CMD.vi"("Cmd String"="Auto-Refresh:Start", "Current Driver Index"=w759) -> ("resulting string"=w765:string)  [unwired: 9 in]
            n343 = call-poly "Enqueue Message.vi"("Message Data"=w761, "Message"="Stop Time", "Message Queue"=w760) -> ("dup Message Queue"=w757:refnum<queue>)  [unwired: 7 in, 1 out]
            n344 = call-poly "Enqueue Message.vi"("Message"=w770, "Message Queue"=w767) -> ("dup Message Queue"=w764:refnum<queue>)  [unwired: 8 in, 1 out]
            n345 = call-poly "Enqueue Message.vi"("Message"=w765, "Message Queue"=w764) -> ()  [unwired: 8 in, 2 out]
            n346 = call-poly "Enqueue Message.vi"("Message"="Open Log File", "Message Queue"=w757) -> ()  [unwired: 8 in, 2 out]
          }
        }
        n347 = Replace Array Subset(array=w719, new element=w718, index=w724) -> (w727:T2[])
      }
      event "Zero Encoder": Value Change {
        n348 = event-data() -> ()  [unwired: 1 in, 6 out]
        n349 = Index Array(array=w773, index=w772) -> (element=w778:T2)
        n350 = Unbundle By Name(w778) -> ("HW Position"=w775:i32)
        n351 = Decrement(x=w775) -> (x-1=w774:i32)
        n352 = call "Driver Parse CMD.vi"("Cmd String"="Encoder Zero", "Current Driver Index"=w774) -> ("resulting string"=w777:string)  [unwired: 9 in]
        n353 = call-poly "Enqueue Message.vi"("Message"=w777, "Message Queue"=w771) -> ()  [unwired: 8 in, 2 out]
      }
      event "Write Digital Out": Value Change {
        # "Copiar de \"Sync DO\""
        n354 = event-data() -> ()  [unwired: 1 in, 6 out]
        n355 = Reshape Array("Output Control", 16 ("dimension size")) -> (w787:bool[])
        n356 = Boolean Array To Number(Boolean array=w787) -> (number=w786:u32)
        n357 = Index Array(array=w793, index=w792) -> (element=w791:T2)
        n358 = To Variant(anything=w786) -> (Variant=w785:variant)
        n359 = Unbundle By Name(w791) -> ("HW Position"=w782:i32)
        n360 = Decrement(x=w782) -> (x-1=w781:i32)
        n361 = call "Driver Parse CMD.vi"("Cmd String"="Digital Out Write", "Current Driver Index"=w781) -> ("resulting string"=w790:string)  [unwired: 9 in]
        n362 = call-poly "Enqueue Message.vi"("Message Data"=w785, "Message"=w790, "Message Queue"=w783) -> ()  [unwired: 7 in, 2 out]
      }
      event "Async ACQ": Value Change {
        n363 = event-data() -> ()  [unwired: 1 in, 6 out]
        n364 = Index Array(array=w801, index=w800) -> (element=w804:T2)
        n365 = Unbundle By Name(w804) -> ("HW Position"=w798:i32)
        n366 = Add(x=w798, y=4) -> (x+y=w797:i32)
        n367 = call "Driver Parse CMD.vi"("Cmd String"="Auto-Cycle", "Current Driver Index"=w797) -> ("resulting string"=w803:string)  [unwired: 9 in]
        n368 = call-poly "Enqueue Message.vi"("Message"=w803, "Message Queue"=w799) -> ()  [unwired: 8 in, 2 out]
      }
      event "Async Zero": Value Change {
        n369 = event-data() -> ()  [unwired: 1 in, 6 out]
        n370 = Index Array(array=w812, index=w811) -> (element=w815:T2)
        n371 = Unbundle By Name(w815) -> ("HW Position"=w809:i32)
        n372 = Add(x=w809, y=4) -> (x+y=w808:i32)
        n373 = call "Driver Parse CMD.vi"("Cmd String"="Auto-Zero", "Current Driver Index"=w808) -> ("resulting string"=w814:string)  [unwired: 9 in]
        n374 = call-poly "Enqueue Message.vi"("Message"=w814, "Message Queue"=w810) -> ()  [unwired: 8 in, 2 out]
      }
      event "Async Action 1": Value Change {
        n375 = event-data() -> ()  [unwired: 1 in, 6 out]
        n376 = Index Array(array=w823, index=w822) -> (element=w826:T2)
        n377 = Unbundle By Name(w826) -> ("HW Position"=w820:i32)
        n378 = Add(x=w820, y=4) -> (x+y=w819:i32)
        n379 = call "Driver Parse CMD.vi"("Cmd String"="Action:1", "Current Driver Index"=w819) -> ("resulting string"=w825:string)  [unwired: 9 in]
        n380 = call-poly "Enqueue Message.vi"("Message"=w825, "Message Queue"=w821) -> ()  [unwired: 8 in, 2 out]
      }
      event "Async Action 2": Value Change {
        n381 = event-data() -> ()  [unwired: 1 in, 6 out]
        n382 = Index Array(array=w834, index=w833) -> (element=w837:T2)
        n383 = Unbundle By Name(w837) -> ("HW Position"=w831:i32)
        n384 = Add(x=w831, y=4) -> (x+y=w830:i32)
        n385 = call "Driver Parse CMD.vi"("Cmd String"="Action:2", "Current Driver Index"=w830) -> ("resulting string"=w836:string)  [unwired: 9 in]
        n386 = call-poly "Enqueue Message.vi"("Message"=w836, "Message Queue"=w832) -> ()  [unwired: 8 in, 2 out]
      }
    }
  }
  n387 = Unbundle By Name(w5) -> ("Notifiers.Acquisition"=w28:T13)
  n388 = Unbundle By Name(w5) -> ("Notifiers.Control"=w27:T14)
  n389 = Unbundle By Name(w4) -> ("HAL"=w110:refnum<queue>)
  n390 = Unbundle By Name(w5) -> ("Queues"=w7:T15)
  n391 = Unbundle By Name(w27) -> ("CTRL HWSync1"=w33:refnum<notifier>, "CTRL HWSync2"=w32:refnum<notifier>, "CTRL HWSync3"=w31:refnum<notifier>, "CTRL HWSync4"=w30:refnum<notifier>, "CTRL HWSync5"=w29:refnum<notifier>)
  n392 = Unbundle By Name(w28) -> ("ACQ HWSync1"=w38:refnum<notifier>, "ACQ HWSync2"=w37:refnum<notifier>, "ACQ HWSync3"=w36:refnum<notifier>, "ACQ HWSync4"=w35:refnum<notifier>, "ACQ HWSync5"=w34:refnum<notifier>)
  n393 = Initialize Array(w68, 5 ("dimension size")) -> (w66:T1[])
  n394 = Initialize Array(timestamp(-75600 s since 1904-01-01) ("current time"), 5 ("dimension size")) -> (w11:timestamp[])
  n395 = Cluster To Array(cluster=w7) -> (array=w6:refnum<queue>[])
  n396 = Unbundle By Name(w4) -> ("MATH"=w14:refnum<queue>)
  n397 = while {
    tunnel: w38 -> [w1054]
    tunnel: w24 -> [w1048]
    tunnel: w37 -> [w1039]
    tunnel: w36 -> [w1038]
    tunnel: w35 -> [w1037]
    tunnel: w34 -> [w1036]
    tunnel: w3 -> [w910]
    tunnel: w33 -> [w1012]
    tunnel: w32 -> [w1011]
    tunnel: w31 -> [w1010]
    tunnel: w30 -> [w1009]
    tunnel: w29 -> [w1008]
    tunnel: w26 -> [w989]
    tunnel: w23 -> [w932]
    tunnel: w22 -> [w931]
    tunnel: w21 -> [w930]
    tunnel: w20 -> [w929]
    tunnel: w19 -> [w928]
    tunnel: w18 -> [w927]
    tunnel: w17 -> [w926]
    tunnel: w16 -> [w925]
    tunnel: w15 -> [w924]
    stop <- w1049 continue-if-true
    w842 = sgl[] [] ("s? t:f")
    w923 = 200  # Timeout(ms)
    # "Display Loop"
    n398 = call "Wait on Async ACQ Notification.vi"("error in (no error)"=w910, "timeout in ms (-1)"=w923, "Async ACQ Notifier in"=w989) -> ("timed out?"=w985:bool, "Async ACQ"=w987:T16)  [unwired: 5 in, 2 out]
    n399 = call "Wait on Async ACQ Notification.vi"("error in (no error)"=w910, "timeout in ms (-1)"=w923, "Async ACQ Notifier in"=w932) -> ("timed out?"=w968:bool, "Async ACQ"=w966:T16)  [unwired: 5 in, 2 out]
    n400 = call "Wait on Async ACQ Notification.vi"("error in (no error)"=w910, "timeout in ms (-1)"=w923, "Async ACQ Notifier in"=w931) -> ("timed out?"=w961:bool, "Async ACQ"=w963:T16)  [unwired: 5 in, 2 out]
    n401 = call "Wait on Async ACQ Notification.vi"("error in (no error)"=w910, "timeout in ms (-1)"=w923, "Async ACQ Notifier in"=w930) -> ("timed out?"=w953:bool, "Async ACQ"=w955:T16)  [unwired: 5 in, 2 out]
    n402 = call "Wait on Async ACQ Notification.vi"("error in (no error)"=w910, "timeout in ms (-1)"=w923, "Async ACQ Notifier in"=w929) -> ("timed out?"=w960:bool, "Async ACQ"=w958:T16)  [unwired: 5 in, 2 out]
    n403 = call "Wait on Async ACQ Notification.vi"("error in (no error)"=w910, "timeout in ms (-1)"=w923, "Async ACQ Notifier in"=w928) -> ("timed out?"=w949:bool, "Async ACQ"=w951:T16)  [unwired: 5 in, 2 out]
    n404 = call "Wait on Async ACQ Notification.vi"("error in (no error)"=w910, "timeout in ms (-1)"=w923, "Async ACQ Notifier in"=w927) -> ("timed out?"=w936:bool, "Async ACQ"=w934:T16)  [unwired: 5 in, 2 out]
    n405 = call "Wait on Async ACQ Notification.vi"("error in (no error)"=w910, "timeout in ms (-1)"=w923, "Async ACQ Notifier in"=w926) -> ("timed out?"=w944:bool, "Async ACQ"=w942:T16)  [unwired: 5 in, 2 out]
    n406 = call "Wait on Async ACQ Notification.vi"("error in (no error)"=w910, "timeout in ms (-1)"=w923, "Async ACQ Notifier in"=w925) -> ("timed out?"=w937:bool, "Async ACQ"=w939:T16)  [unwired: 5 in, 2 out]
    n407 = call "Wait on Async ACQ Notification.vi"("error in (no error)"=w910, "timeout in ms (-1)"=w923, "Async ACQ Notifier in"=w924) -> ("timed out?"=w948:bool, "Async ACQ"=w946:T16)  [unwired: 5 in, 2 out]
    n408 = call "Wait on ACQ Notification.vi"("error in (no error)"=w910, "timeout in ms (-1)"=w923, "ACQ Data Notifier in"=w1054) -> ("timed out?"=w905:bool, "1 Sample"=w909:T17)  [unwired: 5 in, 2 out]
    n409 = call "Wait on ACQ Notification.vi"("error in (no error)"=w910, "timeout in ms (-1)"=w923, "ACQ Data Notifier in"=w1039) -> ("timed out?"=w896:bool, "1 Sample"=w897:T17)  [unwired: 5 in, 2 out]
    n410 = call "Wait on ACQ Notification.vi"("error in (no error)"=w910, "timeout in ms (-1)"=w923, "ACQ Data Notifier in"=w1038) -> ("timed out?"=w891:bool, "1 Sample"=w892:T17)  [unwired: 5 in, 2 out]
    n411 = call "Wait on ACQ Notification.vi"("error in (no error)"=w910, "timeout in ms (-1)"=w923, "ACQ Data Notifier in"=w1037) -> ("timed out?"=w886:bool, "1 Sample"=w887:T17)  [unwired: 5 in, 2 out]
    n412 = call "Wait on ACQ Notification.vi"("error in (no error)"=w910, "timeout in ms (-1)"=w923, "ACQ Data Notifier in"=w1036) -> ("timed out?"=w881:bool, "1 Sample"=w882:T17)  [unwired: 5 in, 2 out]
    n413 = call "Wait on CTRL Notification.vi"("error in (no error)"=w910, "timeout in ms (-1)"=w923, "CTRL Data Notifier in"=w1012) -> ("timed out?"=w901:bool, "Control Data"=w902:T18)  [unwired: 5 in, 2 out]
    n414 = call "Wait on CTRL Notification.vi"("error in (no error)"=w910, "timeout in ms (-1)"=w923, "CTRL Data Notifier in"=w1011) -> ("timed out?"=w876:bool, "Control Data"=w877:T18)  [unwired: 5 in, 2 out]
    n415 = call "Wait on CTRL Notification.vi"("error in (no error)"=w910, "timeout in ms (-1)"=w923, "CTRL Data Notifier in"=w1010) -> ("timed out?"=w870:bool, "Control Data"=w872:T18)  [unwired: 5 in, 2 out]
    n416 = call "Wait on CTRL Notification.vi"("error in (no error)"=w910, "timeout in ms (-1)"=w923, "CTRL Data Notifier in"=w1009) -> ("timed out?"=w866:bool, "Control Data"=w867:T18)  [unwired: 5 in, 2 out]
    n417 = call "Wait on CTRL Notification.vi"("error in (no error)"=w910, "timeout in ms (-1)"=w923, "CTRL Data Notifier in"=w1008) -> ("timed out?"=w861:bool, "Control Data"=w862:T18)  [unwired: 5 in, 2 out]
    n418 = Unbundle By Name(w902) -> ("DO"=w903:bool[])
    n419 = Unbundle By Name(w877) -> ("DO"=w879:bool[])
    n420 = Unbundle By Name(w872) -> ("DO"=w873:bool[])
    n421 = Unbundle By Name(w867) -> ("DO"=w869:bool[])
    n422 = Unbundle By Name(w862) -> ("DO"=w863:bool[])
    n423 = local read "Enable Waveforms"() -> (w843:u32)
    n424 = Wait on Occurrence(1:FALSE ("ignore previous (T)"), 2:w1048, 3:w923) -> (0:w1049:bool)
    n425 = Unbundle By Name(w909) -> ("TDX"=w908:sgl[])
    n426 = Unbundle By Name(w897) -> ("TDX"=w898:sgl[])
    n427 = Unbundle By Name(w892) -> ("TDX"=w894:sgl[])
    n428 = Unbundle By Name(w887) -> ("TDX"=w888:sgl[])
    n429 = Unbundle By Name(w882) -> ("TDX"=w884:sgl[])
    n430 = Empty Array?(array=w903) -> (empty?=w904:bool)
    n431 = Empty Array?(array=w879) -> (empty?=w878:bool)
    n432 = Empty Array?(array=w873) -> (empty?=w874:bool)
    n433 = Empty Array?(array=w869) -> (empty?=w868:bool)
    n434 = Empty Array?(array=w863) -> (empty?=w864:bool)
    n435 = Empty Array?(array=w908) -> (empty?=w907:bool)
    n436 = Empty Array?(array=w898) -> (empty?=w899:bool)
    n437 = Empty Array?(array=w894) -> (empty?=w893:bool)
    n438 = Empty Array?(array=w888) -> (empty?=w889:bool)
    n439 = Empty Array?(array=w884) -> (empty?=w883:bool)
    n440 = Or(x=w904, y=w901) -> (x .or. y?=w900:bool)
    n441 = Or(x=w878, y=w876) -> (x .or. y?=w875:bool)
    n442 = Or(x=w874, y=w870) -> (x .or. y?=w871:bool)
    n443 = Or(x=w868, y=w866) -> (x .or. y?=w865:bool)
    n444 = Or(x=w864, y=w861) -> (x .or. y?=w860:bool)
    n445 = Or(x=w907, y=w905) -> (x .or. y?=w906:bool)
    n446 = Or(x=w899, y=w896) -> (x .or. y?=w895:bool)
    n447 = Or(x=w893, y=w891) -> (x .or. y?=w890:bool)
    n448 = Or(x=w889, y=w886) -> (x .or. y?=w885:bool)
    n449 = Or(x=w883, y=w881) -> (x .or. y?=w880:bool)
    n450 = feedback #2(w987) -> (w988:T16)
    n451 = Select(t=w988, s=w985, f=w987) -> (s? t:f=w986:T16)
    n452 = feedback-in #2(w986) -> ()
    n453 = feedback #3(w966) -> (w965:T16)
    n454 = Select(t=w965, s=w968, f=w966) -> (s? t:f=w967:T16)
    n455 = feedback-in #3(w967) -> ()
    n456 = feedback #4(w963) -> (w964:T16)
    n457 = Select(t=w964, s=w961, f=w963) -> (s? t:f=w962:T16)
    n458 = feedback-in #4(w962) -> ()
    n459 = feedback #5(w955) -> (w956:T16)
    n460 = Select(t=w956, s=w953, f=w955) -> (s? t:f=w954:T16)
    n461 = feedback-in #5(w954) -> ()
    n462 = feedback #6(w958) -> (w957:T16)
    n463 = Select(t=w957, s=w960, f=w958) -> (s? t:f=w959:T16)
    n464 = feedback-in #6(w959) -> ()
    n465 = feedback #7(w951) -> (w952:T16)
    n466 = Select(t=w952, s=w949, f=w951) -> (s? t:f=w950:T16)
    n467 = feedback-in #7(w950) -> ()
    n468 = feedback #8(w934) -> (w933:T16)
    n469 = Select(t=w933, s=w936, f=w934) -> (s? t:f=w935:T16)
    n470 = feedback-in #8(w935) -> ()
    n471 = feedback #9(w942) -> (w941:T16)
    n472 = Select(t=w941, s=w944, f=w942) -> (s? t:f=w943:T16)
    n473 = feedback-in #9(w943) -> ()
    n474 = feedback #10(w939) -> (w940:T16)
    n475 = Select(t=w940, s=w937, f=w939) -> (s? t:f=w938:T16)
    n476 = feedback-in #10(w938) -> ()
    n477 = feedback #11(w946) -> (w945:T16)
    n478 = Select(t=w945, s=w948, f=w946) -> (s? t:f=w947:T16)
    n479 = feedback-in #11(w947) -> ()
    n480 = feedback #12(w902) -> (w1053:T18)
    n481 = Select(t=w1053, s=w900, f=w902) -> (s? t:f=w1052:T18)
    n482 = feedback-in #12(w1052) -> ()
    n483 = feedback #13(w877) -> (w1033:T18)
    n484 = Select(t=w1033, s=w875, f=w877) -> (s? t:f=w1034:T18)
    n485 = feedback-in #13(w1034) -> ()
    n486 = feedback #14(w872) -> (w1032:T18)
    n487 = Select(t=w1032, s=w871, f=w872) -> (s? t:f=w1031:T18)
    n488 = feedback-in #14(w1031) -> ()
    n489 = feedback #15(w867) -> (w1029:T18)
    n490 = Select(t=w1029, s=w865, f=w867) -> (s? t:f=w1030:T18)
    n491 = feedback-in #15(w1030) -> ()
    n492 = feedback #16(w862) -> (w1028:T18)
    n493 = Select(t=w1028, s=w860, f=w862) -> (s? t:f=w1027:T18)
    n494 = feedback-in #16(w1027) -> ()
    n495 = feedback #17(w909) -> (w1051:T17)
    n496 = Select(t=w1051, s=w906, f=w909) -> (s? t:f=w1050:T17)
    n497 = feedback-in #17(w1050) -> ()
    n498 = feedback #18(w897) -> (w1046:T17)
    n499 = Select(t=w1046, s=w895, f=w897) -> (s? t:f=w1047:T17)
    n500 = feedback-in #18(w1047) -> ()
    n501 = feedback #19(w892) -> (w1045:T17)
    n502 = Select(t=w1045, s=w890, f=w892) -> (s? t:f=w1044:T17)
    n503 = feedback-in #19(w1044) -> ()
    n504 = feedback #20(w887) -> (w1042:T17)
    n505 = Select(t=w1042, s=w885, f=w887) -> (s? t:f=w1043:T17)
    n506 = feedback-in #20(w1043) -> ()
    n507 = feedback #21(w882) -> (w1041:T17)
    n508 = Select(t=w1041, s=w880, f=w882) -> (s? t:f=w1040:T17)
    n509 = feedback-in #21(w1040) -> ()
    n510 = Number To Boolean Array(number=w843) -> (Boolean array=w841:bool[])
    n511 = Not(x=w841) -> (.not. x?=w840:bool[])
    n512 = Unbundle By Name(w986) -> ("Data"=w921:sgl[])
    n513 = Unbundle By Name(w967) -> ("Data"=w920:sgl[])
    n514 = Unbundle By Name(w962) -> ("Data"=w919:sgl[])
    n515 = Unbundle By Name(w954) -> ("Data"=w918:sgl[])
    n516 = Unbundle By Name(w959) -> ("Data"=w917:sgl[])
    n517 = Unbundle By Name(w950) -> ("Data"=w916:sgl[])
    n518 = Unbundle By Name(w935) -> ("Data"=w915:sgl[])
    n519 = Unbundle By Name(w943) -> ("Data"=w914:sgl[])
    n520 = Unbundle By Name(w938) -> ("Data"=w913:sgl[])
    n521 = Unbundle By Name(w947) -> ("Data"=w912:sgl[])
    n522 = Unbundle By Name(w1052) -> ("Encoder"=w1035:sgl, "DI"=w1022:bool[], "DO"=w1015:bool[])
    n523 = Unbundle By Name(w1034) -> ("Encoder"=w1026:sgl, "DI"=w1021:bool[], "DO"=w1016:bool[])
    n524 = Unbundle By Name(w1031) -> ("Encoder"=w1025:sgl, "DI"=w1020:bool[], "DO"=w1017:bool[])
    n525 = Unbundle By Name(w1030) -> ("Encoder"=w1024:sgl, "DI"=w1019:bool[], "DO"=w1014:bool[])
    n526 = Unbundle By Name(w1027) -> ("Encoder"=w1023:sgl, "DI"=w1018:bool[], "DO"=w1013:bool[])
    n527 = Unbundle By Name(w1050) -> ("TDX"=w858:sgl[])
    n528 = Unbundle By Name(w1047) -> ("TDX"=w856:sgl[])
    n529 = Unbundle By Name(w1044) -> ("TDX"=w854:sgl[])
    n530 = Unbundle By Name(w1043) -> ("TDX"=w853:sgl[])
    n531 = Unbundle By Name(w1040) -> ("TDX"=w852:sgl[])
    n532 = Index Array(array=w840) -> (element #1=w844:bool, element #2=w845:bool, element #3=w846:bool, element #4=w847:bool, element #5=w848:bool)  [unwired: 5 in]
    n533 = Select(t=w842, s=w844, f=w858) -> (s? t:f=w857:sgl[])
    n534 = Select(t=w842, s=w845, f=w856) -> (s? t:f=w855:sgl[])
    n535 = Select(t=w842, s=w846, f=w854) -> (s? t:f=w849:sgl[])
    n536 = Select(t=w842, s=w847, f=w853) -> (s? t:f=w850:sgl[])
    n537 = Select(t=w842, s=w848, f=w852) -> (s? t:f=w851:sgl[])
    n538 = local read "HW Position"() -> (w979:i32)
    n539 = Build Array(w921, w920, w919, w918, w917, w916, w915, w914, w913, w912) -> (w922:sgl[][])
    n540 = Array Size(array=w857) -> (size(s)=w1007:i32)
    n541 = Build Array(w1035, w1026, w1025, w1024, w1023) -> (w982:sgl[])
    n542 = Build Array(w1022, w1021, w1020, w1019, w1018) -> (w980:bool[][])
    n543 = Build Array(w1015, w1016, w1017, w1014, w1013) -> (w978:bool[][])
    n544 = Initialize Array(sgl 0.0 ("element"), w1007) -> (w1005:sgl[])
    n545 = Decrement(x=w979) -> (x-1=w977:i32)
    n546 = Build Array (concatenate)(w1005, w855) -> (w1001:sgl[])
    n547 = Array Size(array=w1001) -> (size(s)=w1002:i32)
    n548 = Initialize Array(sgl 0.0 ("element"), w1002) -> (w1004:sgl[])
    n549 = Build Array (concatenate)(w1004, w849) -> (w998:sgl[])
    n550 = Array Size(array=w998) -> (size(s)=w997:i32)
    n551 = Initialize Array(sgl 0.0 ("element"), w997) -> (w999:sgl[])
    n552 = Build Array (concatenate)(w999, w850) -> (w992:sgl[])
    n553 = Array Size(array=w992) -> (size(s)=w996:i32)
    n554 = Initialize Array(sgl 0.0 ("element"), w996) -> (w995:sgl[])
    n555 = Build Array (concatenate)(w995, w851) -> (w993:sgl[])
    n556 = Build Array(w857, w855, w849, w850, w851) -> (w991:sgl[][])
    n557 = Number To Fractional String(number=w922, precision (6)=i16 3) -> (F-format string=→"Tabla Med Async":string[][])  [unwired: 2 in]
    n558 = Index Array(array=w982, index=w977) -> (element=→"Encoder":sgl)
    n559 = Index Array(array=w980, index (row)=w977) -> (element=w976:bool[])  [unwired: 1 in]
    n560 = Index Array(array=w978, index (row)=w977) -> (element=w971:bool[])  [unwired: 1 in]
    n561 = Number To Fractional String(number=w991) -> (F-format string=→"Tabla TDX":string[][])  [unwired: 3 in]
    n562 = Build Array(w857, w1001, w998, w992, w993) -> (→"Waveform Graph":sgl[][])
    n563 = Reshape Array(w976, 2 ("dimension size"), 16 ("dimension size")) -> (→"Sync DI":bool[][])
    n564 = Reshape Array(w971, 2 ("dimension size"), 16 ("dimension size")) -> (→"Sync DO":bool[][])
  }
  n565 = Initialize Array(w10, 5 ("dimension size")) -> (w8:T1[])
  n566 = while {
    tunnel: w110 -> [w1069]
    tunnel: w3 -> [w1068]
    tunnel: [w1060] -> w46
    tunnel: w4 -> [w1059]
    shift-right: [w1056] -> _
    shift-left: w66 -> [w1057]
    tunnel: w44 -> [w1055]
    stop <- w1064 stop-if-true
    # "CMD"
    # "HAL Message Switch Loop"
    n567 = call "Dequeue Message.vi"("error in (no error)"=w1068, "Message Queue"=w1069) -> ("error out"=w1067:errorcluster, "Message Data"=w1066:variant, "Message"=w1063:string, "dup Message Queue"=w1065:refnum<queue>)  [unwired: 6 in]
    n568 = Match Pattern(string=w1063, regular expression=":") -> (before substring=w1061:string, after substring=w1058:string)  [unwired: 1 in, 2 out]
    n569 = case shown="\"ERROR\"" w1061 {
      tunnel: w1067 -> [w1071 w1078 w1103 w1127 w1140 w1159 w1182 w1193 w1230]
      tunnel: w1066 -> [_ _ w1101 w1125 w1139 w1158 w1181 w1201 w1235]
      tunnel: w1065 -> [_ _ _ _ _ _ _ _ _]
      tunnel: [_ TRUE _ _ _ _ _ _ _] -> w1064
      tunnel: [w1071 w1077 w1102 w1126 w1138 w1159 w1174 w1200 w1234] -> w1060
      tunnel: w1059 -> [_ w1075 w1100 w1124 _ _ w1173 _ _]
      tunnel: w1058 -> [_ _ w1093 w1118 w1131 w1162 _ w1187 w1217]
      tunnel: w1057 -> [w1070 w1072 w1085 w1104 w1132 w1160 w1176 w1192 w1229]
      tunnel: [w1070 w1072 w1085 w1104 w1132 w1160 w1170 w1192 w1229] -> w1056
      tunnel: w1055 -> [_ _ _ _ _ w1157 _ _ _]
      frame Default {
      }
      frame "EXIT" {
        n570 = Cluster To Array(cluster=w1075) -> (array=w1074:refnum<queue>[])
        n571 = for {
          tunnel: w1074 -> [w1082] mode=indexing
          tunnel: "EXIT" ("regular expression") -> [w1081]
          tunnel: w1078 -> [w1084]
          tunnel: [w1083] -> w1077
          tunnel: TRUE -> [w1080]
          n572 = call-poly "Enqueue Message.vi"("Priority Message? (F)"=w1080, "error in (no error)"=w1084, "Message"=w1081, "Message Queue"=w1082) -> ("error out"=w1083:errorcluster)  [unwired: 6 in, 1 out]
        }
      }
      frame "HWSync" {
        # "\"<Tipo HW>:<Indice HW>:<Msje>\" ; <Datos Msje>"
        n573 = Unbundle By Name(w1100) -> ("HWSync1"=w1096:refnum<queue>, "HWSync2"=w1098:refnum<queue>, "HWSync3"=w1099:refnum<queue>, "HWSync4"=w1097:refnum<queue>, "HWSync5"=w1095:refnum<queue>)
        n574 = Match Pattern(string=w1093, regular expression=":") -> (before substring=w1090:string, after substring=w1088:string)  [unwired: 1 in, 2 out]
        n575 = Bundle("HWSync1"=w1096, "HWSync2"=w1098, "HWSync3"=w1099, "HWSync4"=w1097, "HWSync5"=w1095) -> (w1092:T19)  [unwired: 1 in]
        n576 = Decimal String To Number(string=w1090) -> (number=w1086:i32)  [unwired: 2 in, 1 out]
        n577 = Cluster To Array(cluster=w1092) -> (array=w1091:refnum<queue>[])
        n578 = Decrement(x=w1086) -> (x-1=w1087:i32)
        n579 = Index Array(array=w1091, index=w1087) -> (element=w1089:refnum<queue>)
        n580 = call-poly "Enqueue Message.vi"("error in (no error)"=w1103, "Message Data"=w1101, "Message"=w1088, "Message Queue"=w1089) -> ("error out"=w1102:errorcluster)  [unwired: 6 in, 1 out]
      }
      frame "HWAsync" {
        # "\"<Tipo HW>:<Indice HW>:<Msje>\" ; <Datos Msje>"
        n581 = Match Pattern(string=w1118, regular expression=":") -> (before substring=w1115:string, after substring=w1113:string)  [unwired: 1 in, 2 out]
        n582 = Unbundle By Name(w1124) -> ("HWAsync1"=w1121:refnum<queue>, "HWAsync2"=w1105:refnum<queue>, "HWAsync3"=w1123:refnum<queue>, "HWAsync4"=w1122:refnum<queue>, "HWAsync5"=w1120:refnum<queue>, "HWAsync6"=w1106:refnum<queue>, "HWAsync7"=w1107:refnum<queue>, "HWAsync8"=w1108:refnum<queue>, "HWAsync9"=w1109:refnum<queue>, "HWAsync10"=w1110:refnum<queue>)
        n583 = Decimal String To Number(string=w1115) -> (number=w1111:i32)  [unwired: 2 in, 1 out]
        n584 = Decrement(x=w1111) -> (x-1=w1112:i32)
        n585 = Bundle("HWAsync1"=w1121, "HWAsync2"=w1105, "HWAsync3"=w1123, "HWAsync4"=w1122, "HWAsync5"=w1120, "HWAsync6"=w1106, "HWAsync7"=w1107, "HWAsync8"=w1108, "HWAsync9"=w1109, "HWAsync10"=w1110) -> (w1117:T20)  [unwired: 1 in]
        n586 = Cluster To Array(cluster=w1117) -> (array=w1116:refnum<queue>[])
        n587 = Index Array(array=w1116, index=w1112) -> (element=w1114:refnum<queue>)
        n588 = call-poly "Enqueue Message.vi"("error in (no error)"=w1127, "Message Data"=w1125, "Message"=w1113, "Message Queue"=w1114) -> ("error out"=w1126:errorcluster)  [unwired: 6 in, 1 out]
      }
      frame "ACK" {
        # "\"ACK:<Tipo>:<Indice>\" ; \"<Msje Ejecutado>\""
        n589 = Match Pattern(string=w1131, regular expression=":") -> (before substring=w1135:string, after substring=w1133:string)  [unwired: 1 in, 2 out]
        n590 = Get Date/Time In Seconds() -> (seconds since 1Jan1904=w1130:timestamp)
        n591 = Variant To Data(error in=w1140, type="", Variant=w1139) -> (data=w1137:string, error out=w1138:errorcluster)
        n592 = Format Date/Time String(time format string (%c)="%H:%M:%S%2u -> ", seconds (now)=w1130) -> (date/time string=w1128:string)  [unwired: 1 in]
        n593 = case shown="\"HWAsync\"" w1135 {
          selector: w1135 -> [_ w1144 w1156]
          tunnel: w1137 -> [_ w1142 w1151]
          tunnel: w1133 -> [_ w1143 w1155]
          tunnel: w1128 -> [_ w1141 w1150]
          frame Default {
          }
          frame "HWSync" {
            n594 = Format Into String(format string="(%s%s) OK -> %s%s\\r\\n", w1144, w1143, w1141, w1142) -> (resulting string=w1147:string)  [unwired: 2 in, 1 out]
            n595 = local read "Mensajes para Usuario (Síncronos)"() -> (w1146:string)
            n596 = Concatenate Strings(w1147, w1146) -> (→"Mensajes para Usuario (Síncronos)":string)
          }
          frame "HWAsync" {
            (unwired) "%s:%s -> %s\\r\\n" ("format string")
            n597 = local read "Mensajes para el usuario (Asíncronos)"() -> (w1153:string)
            n598 = Format Into String(format string="(%s%s) OK -> %s%s\\r\\n", w1156, w1155, w1150, w1151) -> (resulting string=w1154:string)  [unwired: 2 in, 1 out]
            n599 = Concatenate Strings(w1154, w1153) -> (→"Mensajes para el usuario (Asíncronos)":string)
          }
        }
      }
      frame "CONFIG" {
        # "\"CONFIG:<Tipo>:<Indice>\" ; <Config Data>"
        n600 = Match Pattern(string=w1162, regular expression=":") -> (before substring=w1163:string, after substring=w1161:string)  [unwired: 1 in, 2 out]
        n601 = case shown="\"HWAsync\"" w1163 {
          tunnel: w1161 -> [_ _ _]
          tunnel: w1158 -> [_ w1165 w1167]
          tunnel: w1157 -> [_ w1166 w1168]
          frame Default {
          }
          frame "HWSync" {
            n602 = Generate User Event(user event=w1166, event data cluster=w1165) -> ()  [unwired: 2 in, 2 out]
          }
          frame "HWAsync" {
            n603 = Generate User Event(user event=w1168, event data cluster=w1167) -> ()  [unwired: 2 in, 2 out]
          }
        }
      }
      frame "Update Driver Config" {
        w1180 = T1 {"HWSync Index"=0, "Driver Name"="", "Channel Mask"=0}  # HAL Config Data
        n604 = Unbundle By Name(w1173) -> ("MATH"=w1172:refnum<queue>)
        n605 = Variant To Data(error in=w1182, type=w1180, Variant=w1181) -> (data=w1177:T1, error out=w1175:errorcluster)
        n606 = Unbundle By Name(w1177) -> ("HWSync Index"=w1179:u32)
        n607 = Decrement(x=w1179) -> (x-1=w1178:u32)
        n608 = Replace Array Subset(array=w1176, new element=w1177, index=w1178) -> (w1170:T1[])
        n609 = To Variant(anything=w1170) -> (Variant=w1171:variant)
        n610 = call-poly "Enqueue Message.vi"("error in (no error)"=w1175, "Message Data"=w1171, "Message"="Update HAL Config" ("regular expression"), "Message Queue"=w1172) -> ("error out"=w1174:errorcluster)  [unwired: 6 in, 1 out]
      }
      frame "ERROR" {
        # "\"ERROR:<Tipo HW>:<Indice HW>\" ; <Error ocurrido>"
        n611 = Match Pattern(string=w1187, regular expression=":") -> (before substring=w1189:string, after substring=w1188:string)  [unwired: 1 in, 2 out]
        n612 = Variant To Data(error in=w1193, type=w1193, Variant=w1201) -> (data=w1183:errorcluster, error out=w1200:errorcluster)
        n613 = Unbundle By Name(w1183) -> ("source"=w1185:string)
        n614 = Match Pattern(string=w1185, regular expression="<ERR>") -> (after substring=w1195:string)  [unwired: 1 in, 3 out]
        n615 = Get Date/Time In Seconds() -> (seconds since 1Jan1904=w1198:timestamp)
        n616 = String Subset(string=w1195, offset (0)=1) -> (substring=w1184:string)  [unwired: 1 in]
        n617 = Format Date/Time String(time format string (%c)="%H:%M:%S%2u -> ", seconds (now)=w1198) -> (date/time string=w1196:string)  [unwired: 1 in]
        n618 = Concatenate Strings(w1196, "<ERR>" ("string"), w1184) -> (w1186:string)
        n619 = case shown="\"HWSync\"" w1189 {
          selector: w1189 -> [_ w1204 w1214]
          tunnel: w1186 -> [_ w1205 w1212]
          tunnel: w1188 -> [_ w1203 w1213]
          frame Default {
          }
          frame "HWSync" {
            n620 = Format Into String(format string="(%s%s) ERROR -> %s\\r\\n", w1204, w1203, w1205) -> (resulting string=w1207:string)  [unwired: 2 in, 1 out]
            n621 = local read "Mensajes para Usuario (Síncronos)"() -> (w1206:string)
            n622 = Concatenate Strings(w1207, w1206) -> (w1202:string)
            n623 = local write "Mensajes para Usuario (Síncronos)"(w1202) -> ()
          }
          frame "HWAsync" {
            (unwired) "(%s%s) ERROR -> %s\\r\\n" ("format string")
            n624 = local read "Mensajes para el usuario (Asíncronos)"() -> (w1210:string)
            n625 = Format Into String(format string="%s:%s -> %s\\r\\n", w1214, w1213, w1212) -> (resulting string=w1211:string)  [unwired: 2 in, 1 out]
            n626 = Concatenate Strings(w1211, w1210) -> (w1209:string)
            n627 = local write "Mensajes para el usuario (Asíncronos)"(w1209) -> ()
          }
        }
      }
      frame "WARNING" {
        # "\"WARNING:<Tipo HW>:<Indice HW>\" ; <Advertencia ocurrida>"
        n628 = Match Pattern(string=w1217, regular expression=":") -> (before substring=w1219:string, after substring=w1218:string)  [unwired: 1 in, 2 out]
        n629 = Variant To Data(error in=w1230, type=w1230, Variant=w1235) -> (data=w1227:errorcluster, error out=w1234:errorcluster)
        n630 = Unbundle By Name(w1227) -> ("code"=w1222:i32, "source"=w1226:string)
        n631 = Match Pattern(string=w1226, regular expression="<ERR>") -> (after substring=w1224:string)  [unwired: 1 in, 3 out]
        n632 = Pick Line(multi-line string=w1224, line index=2) -> (output string=w1223:string)  [unwired: 1 in]
        n633 = Get Date/Time In Seconds() -> (seconds since 1Jan1904=w1233:timestamp)
        n634 = Format Date/Time String(time format string (%c)="%H:%M:%S%2u -> ", seconds (now)=w1233) -> (date/time string=w1231:string)  [unwired: 1 in]
        n635 = Number To Decimal String(number=w1222) -> (decimal integer string=w1228:string)  [unwired: 1 in]
        n636 = Concatenate Strings(w1231, w1223, w1228) -> (w1216:string)
        n637 = case shown="\"HWAsync\"" w1219 {
          selector: w1219 -> [_ w1238 w1248]
          tunnel: w1216 -> [_ w1239 w1246]
          tunnel: w1218 -> [_ w1237 w1247]
          frame Default {
          }
          frame "HWSync" {
            n638 = Format Into String(format string="(%s%s) MSJE -> %s\\r\\n", w1238, w1237, w1239) -> (resulting string=w1241:string)  [unwired: 2 in, 1 out]
            n639 = local read "Mensajes para Usuario (Síncronos)"() -> (w1240:string)
            n640 = Concatenate Strings(w1241, w1240) -> (w1236:string)
            n641 = local write "Mensajes para Usuario (Síncronos)"(w1236) -> ()
          }
          frame "HWAsync" {
            (unwired) "(%s%s) MSJE -> %s\\r\\n" ("format string")
            n642 = local read "Mensajes para el usuario (Asíncronos)"() -> (w1244:string)
            n643 = Format Into String(format string="%s:%s -> %s\\r\\n", w1248, w1247, w1246) -> (resulting string=w1245:string)  [unwired: 2 in, 1 out]
            n644 = Concatenate Strings(w1245, w1244) -> (w1243:string)
            n645 = local write "Mensajes para el usuario (Asíncronos)"(w1243) -> ()
          }
        }
      }
    }
  }
  n646 = while {
    tunnel: w6 -> [w1250]
    tunnel: w14 -> [w1263]
    shift-right: [w1255] -> _
    shift-left: w8 -> [w1257]
    shift-right: [w1253] -> _
    shift-left: w11 -> [w1254]
    tunnel: w3 -> [w1259]
    tunnel: [w1260] -> _
    shift-right: [w1251] -> _
    shift-left: w11 -> [w1252]
    stop <- w1262 stop-if-true
    # "Logging Loop"
    n647 = call "Dequeue Message.vi"("error in (no error)"=w1259, "Message Queue"=w1263) -> ("error out"=w1261:errorcluster, "Message Data"=w1256:variant, "Message"=w1264:string, "dup Message Queue"=w1258:refnum<queue>)  [unwired: 6 in]
    n648 = case shown="\"Start Time\"" w1264 {
      tunnel: w1258 -> [_ _ _ _ _ _]
      tunnel: [_ _ _ _ _ TRUE] -> w1262
      tunnel: w1261 -> [w1268 w1273 w1284 w1294 w1300 w1304]
      tunnel: [w1268 w1272 w1283 w1293 w1300 w1304] -> w1260
      tunnel: w1257 -> [w1267 w1270 w1285 w1295 w1299 w1303]
      tunnel: [w1267 w1269 w1285 w1295 w1299 w1303] -> w1255
      tunnel: w1256 -> [_ w1271 w1282 w1292 _ _]
      tunnel: w1254 -> [w1265 w1275 w1279 w1286 w1298 w1301]
      tunnel: [w1265 w1275 w1277 w1286 w1298 w1301] -> w1253
      tunnel: w1252 -> [w1266 w1274 w1276 w1288 w1297 w1302]
      tunnel: [w1266 w1274 w1276 w1287 w1297 w1302] -> w1251
      tunnel: w1250 -> [_ _ _ _ w1296 _]
      frame Default {
      }
      frame "Update HAL Config" {
        n649 = Variant To Data(error in=w1273, type=w1270, Variant=w1271) -> (data=w1269:T1[], error out=w1272:errorcluster)
      }
      frame "Start Time" {
        n650 = Variant To Data(error in=w1284, type=u32 0, Variant=w1282) -> (data=w1280:u32, error out=w1283:errorcluster)
        n651 = Get Date/Time In Seconds() -> (seconds since 1Jan1904=w1278:timestamp)
        n652 = Replace Array Subset(array=w1279, new element=w1278, index=w1280) -> (w1277:timestamp[])
      }
      frame "Stop Time" {
        n653 = Variant To Data(error in=w1294, type=u32 0, Variant=w1292) -> (data=w1290:u32, error out=w1293:errorcluster)
        n654 = Get Date/Time In Seconds() -> (seconds since 1Jan1904=w1289:timestamp)
        n655 = Replace Array Subset(array=w1288, new element=w1289, index=w1290) -> (w1287:timestamp[])
      }
      frame "Open Log File" {
        n656 = call "CreateLogFile.vi"("Stop Time"=w1297, "Start Time"=w1298, "HAL Config"=w1299, "ACQ Queues"=w1296) -> ()  [unwired: 8 in]
      }
      frame "EXIT" {
      }
    }
  }
  n657 = Unbundle By Name(w5) -> ("Notifiers.Async.ACQ HWAsync10"=w56:refnum<notifier>)
  n658 = Unbundle By Name(w5) -> ("Notifiers.Async.ACQ HWAsync1"=w65:refnum<notifier>)
  n659 = Unbundle By Name(w5) -> ("Notifiers.Async.ACQ HWAsync2"=w64:refnum<notifier>)
  n660 = Unbundle By Name(w5) -> ("Notifiers.Async.ACQ HWAsync3"=w63:refnum<notifier>)
  n661 = Unbundle By Name(w5) -> ("Notifiers.Async.ACQ HWAsync4"=w62:refnum<notifier>)
  n662 = Unbundle By Name(w5) -> ("Notifiers.Async.ACQ HWAsync5"=w61:refnum<notifier>)
  n663 = Unbundle By Name(w5) -> ("Notifiers.Async.ACQ HWAsync6"=w60:refnum<notifier>)
  n664 = Unbundle By Name(w5) -> ("Notifiers.Async.ACQ HWAsync7"=w59:refnum<notifier>)
  n665 = Unbundle By Name(w5) -> ("Notifiers.Async.ACQ HWAsync8"=w58:refnum<notifier>)
  n666 = Unbundle By Name(w5) -> ("Notifiers.Async.ACQ HWAsync9"=w57:refnum<notifier>)
  n667 = Unbundle By Name(w5) -> ("Notifiers.Acquisition.ACQ HWSync1"=w142:refnum<notifier>, "Notifiers.Control.CTRL HWSync1"=w141:refnum<notifier>, "Queues.ACQ HWSync1"=w140:refnum<queue>)
  n668 = Unbundle By Name(w5) -> ("Notifiers.Acquisition.ACQ HWSync2"=w137:refnum<notifier>, "Notifiers.Control.CTRL HWSync2"=w138:refnum<notifier>, "Queues.ACQ HWSync2"=w139:refnum<queue>)
  n669 = Unbundle By Name(w5) -> ("Notifiers.Acquisition.ACQ HWSync3"=w125:refnum<notifier>, "Notifiers.Control.CTRL HWSync3"=w126:refnum<notifier>, "Queues.ACQ HWSync3"=w127:refnum<queue>)
  n670 = Unbundle By Name(w5) -> ("Notifiers.Acquisition.ACQ HWSync4"=w130:refnum<notifier>, "Notifiers.Control.CTRL HWSync4"=w129:refnum<notifier>, "Queues.ACQ HWSync4"=w128:refnum<queue>)
  n671 = Unbundle By Name(w5) -> ("Notifiers.Acquisition.ACQ HWSync5"=w119:refnum<notifier>, "Notifiers.Control.CTRL HWSync5"=w120:refnum<notifier>, "Queues.ACQ HWSync5"=w121:refnum<queue>)
  n672 = Unbundle By Name(w4) -> ("HAL"=w92:refnum<queue>, "HWAsync10"=w93:refnum<queue>)
  n673 = Unbundle By Name(w4) -> ("HAL"=w109:refnum<queue>, "HWAsync1"=w108:refnum<queue>)
  n674 = Unbundle By Name(w4) -> ("HAL"=w104:refnum<queue>, "HWAsync2"=w105:refnum<queue>)
  n675 = Unbundle By Name(w4) -> ("HAL"=w103:refnum<queue>, "HWAsync3"=w102:refnum<queue>)
  n676 = Unbundle By Name(w4) -> ("HAL"=w98:refnum<queue>, "HWAsync4"=w99:refnum<queue>)
  n677 = Unbundle By Name(w4) -> ("HAL"=w97:refnum<queue>, "HWAsync5"=w96:refnum<queue>)
  n678 = Unbundle By Name(w4) -> ("HAL"=w80:refnum<queue>, "HWAsync6"=w81:refnum<queue>)
  n679 = Unbundle By Name(w4) -> ("HAL"=w85:refnum<queue>, "HWAsync7"=w84:refnum<queue>)
  n680 = Unbundle By Name(w4) -> ("HAL"=w86:refnum<queue>, "HWAsync8"=w87:refnum<queue>)
  n681 = Unbundle By Name(w4) -> ("HAL"=w91:refnum<queue>, "HWAsync9"=w90:refnum<queue>)
  n682 = Unbundle By Name(w4) -> ("HAL"=w145:refnum<queue>, "HWSync1"=w144:refnum<queue>)
  n683 = Unbundle By Name(w4) -> ("HAL"=w134:refnum<queue>, "HWSync2"=w135:refnum<queue>)
  n684 = Unbundle By Name(w4) -> ("HAL"=w122:refnum<queue>, "HWSync3"=w123:refnum<queue>)
  n685 = Unbundle By Name(w4) -> ("HAL"=w133:refnum<queue>, "HWSync4"=w132:refnum<queue>)
  n686 = Unbundle By Name(w4) -> ("HAL"=w116:refnum<queue>, "HWSync5"=w117:refnum<queue>)
  n687 = call "HWSyncLoop.vi"("HAL"=w145, "Index"=u32 1 ("Num of Loop"), "HWSync"=w144, "error in"=w3, "ACQ Data Queue"=w140, "CTRL Data Notifier"=w141, "ACQ Data Notifier"=w142) -> ("error out"=w115:errorcluster)  [unwired: 4 in]
  n688 = call "HWSyncLoop.vi"("HAL"=w134, "Index"=u32 2 ("Num of Loop"), "HWSync"=w135, "error in"=w3, "ACQ Data Queue"=w139, "CTRL Data Notifier"=w138, "ACQ Data Notifier"=w137) -> ("error out"=w114:errorcluster)  [unwired: 4 in]
  n689 = call "HWSyncLoop.vi"("HAL"=w122, "Index"=u32 3 ("Num of Loop"), "HWSync"=w123, "error in"=w3, "ACQ Data Queue"=w127, "CTRL Data Notifier"=w126, "ACQ Data Notifier"=w125) -> ("error out"=w113:errorcluster)  [unwired: 4 in]
  n690 = call "HWSyncLoop.vi"("HAL"=w133, "Index"=u32 4 ("Num of Loop"), "HWSync"=w132, "error in"=w3, "ACQ Data Queue"=w128, "CTRL Data Notifier"=w129, "ACQ Data Notifier"=w130) -> ("error out"=w112:errorcluster)  [unwired: 4 in]
  n691 = call "HWSyncLoop.vi"("HAL"=w116, "Index"=u32 5 ("Num of Loop"), "HWSync"=w117, "error in"=w3, "ACQ Data Queue"=w121, "CTRL Data Notifier"=w120, "ACQ Data Notifier"=w119) -> ("error out"=w111:errorcluster)  [unwired: 4 in]
  n692 = call "HWAsyncLoop.vi"("HAL"=w109, "Index"=u32 1, "HWAsync"=w108, "error in"=w3, "Async ACQ Notifier in"=w65) -> ("error out"=w79:errorcluster)  [unwired: 6 in]
  n693 = call "HWAsyncLoop.vi"("HAL"=w104, "Index"=u32 2, "HWAsync"=w105, "error in"=w3, "Async ACQ Notifier in"=w64) -> ("error out"=w77:errorcluster)  [unwired: 6 in]
  n694 = call "HWAsyncLoop.vi"("HAL"=w103, "Index"=u32 3, "HWAsync"=w102, "error in"=w3, "Async ACQ Notifier in"=w63) -> ("error out"=w76:errorcluster)  [unwired: 6 in]
  n695 = call "HWAsyncLoop.vi"("HAL"=w98, "Index"=u32 4, "HWAsync"=w99, "error in"=w3, "Async ACQ Notifier in"=w62) -> ("error out"=w75:errorcluster)  [unwired: 6 in]
  n696 = call "HWAsyncLoop.vi"("HAL"=w97, "Index"=u32 5, "HWAsync"=w96, "error in"=w3, "Async ACQ Notifier in"=w61) -> ("error out"=w74:errorcluster)  [unwired: 6 in]
  n697 = call "HWAsyncLoop.vi"("HAL"=w80, "Index"=u32 6, "HWAsync"=w81, "error in"=w3, "Async ACQ Notifier in"=w60) -> ("error out"=w73:errorcluster)  [unwired: 6 in]
  n698 = call "HWAsyncLoop.vi"("HAL"=w85, "Index"=u32 7, "HWAsync"=w84, "error in"=w3, "Async ACQ Notifier in"=w59) -> ("error out"=w72:errorcluster)  [unwired: 6 in]
  n699 = call "HWAsyncLoop.vi"("HAL"=w86, "Index"=u32 8, "HWAsync"=w87, "error in"=w3, "Async ACQ Notifier in"=w58) -> ("error out"=w71:errorcluster)  [unwired: 6 in]
  n700 = call "HWAsyncLoop.vi"("HAL"=w91, "Index"=u32 9, "HWAsync"=w90, "error in"=w3, "Async ACQ Notifier in"=w57) -> ("error out"=w70:errorcluster)  [unwired: 6 in]
  n701 = call "HWAsyncLoop.vi"("HAL"=w92, "Index"=u32 10, "HWAsync"=w93, "error in"=w3, "Async ACQ Notifier in"=w56) -> ("error out"=w69:errorcluster)  [unwired: 6 in]
  n702 = Merge Errors(w79, w77, w76, w75, w74, w73, w72, w71, w70, w69) -> (w78:errorcluster)
  n703 = Destroy User Event(user event=w44, error in=w46) -> (error out=w45:errorcluster)
  n704 = Set Occurrence(w25) -> ()
  n705 = Merge Errors(w115, w114, w113, w112, w111, w78) -> (w55:errorcluster)
  n706 = Merge Errors(w3, w45, w55) -> (w148:errorcluster)
  n707 = call "Destroy All Data Queues.vi"("Error In"=w148, "WINFAS 2 Data Queue.lvlib:All Data Queues Cluster"=w5) -> ("Error Out"=w147:errorcluster)  [unwired: 9 in]
  n708 = call "Destroy All Message Queues.vi"("error in (no error)"=w147, "Message Queues Out"=w4) -> ("error out"=w146:errorcluster)  [unwired: 9 in]
  n709 = property class="App"(error in=w146) -> ("App.Kind"=w150:T21)  [unwired: 1 in, 2 out]
  n710 = case shown="\"Development System\"" w150 {
    tunnel: [TRUE FALSE TRUE] -> w149
    tunnel: [w1306 w1320 w1326] -> _
    frame "invalid app kind", Default {
      n711 = property class="VI"() -> (error out=w1307:errorcluster, "Panel"=w1317:refnum<vi>)  [unwired: 2 in, 1 out]
      n712 = property class="Pnl"(reference=w1317, error in=w1307) -> (error out=w1308:errorcluster, "AllObjs[]"=w1316:refnum<vi>[])  [unwired: 1 out]
      n713 = control-ref of="This VI"() -> (w1314:refnum<vi>)
      n714 = Close Reference(reference=w1316, error in (no error)=w1308) -> (error out=w1313:errorcluster)
      n715 = invoke class="VI" method="FP.Close"(reference=w1314, error in=w1313) -> (reference out=w1312:refnum<vi>, error out=w1311:errorcluster)  [unwired: 1 in, 1 out]
      n716 = invoke class="VI" method="Abort VI"(reference=w1312, error in=w1311) -> (reference out=w1309:refnum<vi>, error out=w1310:errorcluster)  [unwired: 1 in, 1 out]
      n717 = Close Reference(reference=w1309, error in (no error)=w1310) -> (error out=w1318:errorcluster)
      n718 = control-ref of="This Application"() -> (w1319:refnum<vi>)
      n719 = Close Reference(reference=w1319, error in (no error)=w1318) -> (error out=w1306:errorcluster)
    }
    frame "Development System" {
      n720 = property class="VI"() -> (error out=w1321:errorcluster, "Panel"=w1325:refnum<vi>)  [unwired: 2 in, 1 out]
      n721 = property class="Pnl"(reference=w1325, error in=w1321) -> (error out=w1322:errorcluster, "AllObjs[]"=w1324:refnum<vi>[])  [unwired: 1 out]
      n722 = Close Reference(reference=w1324, error in (no error)=w1322) -> (error out=w1320:errorcluster)
    }
    frame "Run Time System" {
      n723 = property class="VI"() -> (error out=w1327:errorcluster, "Panel"=w1337:refnum<vi>)  [unwired: 2 in, 1 out]
      n724 = property class="Pnl"(reference=w1337, error in=w1327) -> (error out=w1328:errorcluster, "AllObjs[]"=w1336:refnum<vi>[])  [unwired: 1 out]
      n725 = control-ref of="This VI"() -> (w1334:refnum<vi>)
      n726 = Close Reference(reference=w1336, error in (no error)=w1328) -> (error out=w1333:errorcluster)
      n727 = invoke class="VI" method="FP.Close"(reference=w1334, error in=w1333) -> (reference out=w1332:refnum<vi>, error out=w1331:errorcluster)  [unwired: 1 in, 1 out]
      n728 = invoke class="VI" method="Abort VI"(reference=w1332, error in=w1331) -> (reference out=w1329:refnum<vi>, error out=w1330:errorcluster)  [unwired: 1 in, 1 out]
      n729 = Close Reference(reference=w1329, error in (no error)=w1330) -> (error out=w1338:errorcluster)
      n730 = control-ref of="This Application"() -> (w1339:refnum<vi>)
      n731 = Close Reference(reference=w1339, error in (no error)=w1338) -> (error out=w1326:errorcluster)
    }
  }
  n732 = Quit LabVIEW(quit? (T)=w149) -> ()
